vi "4Pi Objective Lock - EMBL_v2.vi"(7 "Calling VI Ref":refnum<vi>) -> ()   [LabVIEW 2021]
uses:
  <vilib>/Utility/miscctls.llb/LVPointTypeDef.ctl
  4Pi Objective Lock Type Defs/4Pi Obj Lock - Notifier Type.ctl
  4Pi Objective Lock Type Defs/4Pi Obj Lock - Actions.ctl
  <vilib>/vision/Image Controls.llb/IMAQ Image.ctl
  4Pi Objective Lock Type Defs/4Pi Obj Lock - Lock Settings.ctl
  Hardware Configuration/Hardware Configuration Controls/Device Type.ctl
  Hardware Configuration/Hardware Configuration Controls/Device Function.ctl
  4Pi Objective Lock Type Defs/4Pi Obj Lock - Camera Settings.ctl
  Device Library/Cameras/Camera Controls/Generic Camera ROI.ctl
  Device Library/Cameras/Camera Controls/Generic Camera Actions.ctl
  Device Library/Stages/Stages Controls/Stage Actions.ctl
  <vilib>/addons/control/pid/pid.llb/PID (DBL Array).vi
  <vilib>/addons/control/pid/pid.llb/PID (DBL).vi
  <vilib>/addons/control/pid/NI_PID_pid.lvlib
  <vilib>/vision/NI_Vision_Development_Module.lvlib
panel:
  out "dz (µm)":dbl format="%.2f"
  out "dxy (px)":dbl[](array[numeric])
  in  "Main Tab":T1(tab)
  out "CC Max Value":dbl=1.0 format="%.3g"
  out "dt z (s)":dbl format="%.3f"
  out "CC Max":cluster{"pixel size (µm)":dbl}(graph)
  out "Z Move":bool
  out "XY Move":bool
  out "Measured X Position (px)":dbl=1.0 format="%.3g"
  out "Measured Y Position (px)":dbl=1.0 format="%.3g"
  out "Measured sx/sy":dbl=1.0 format="%.3g"
  out "Target X Position (px)":dbl=1.0 format="%.3g"
  out "Target Y Position (px)":dbl=1.0 format="%.3g"
  out "Target sx/sy":dbl=1.0 format="%.3g"
  out "Z Axis Position (µm)":dbl=1.0 format="%.4g"
  out "Y Axis Position (µm)":dbl=1.0 format="%.2g"
  out "X Axis Position (µm)":dbl=1.0 format="%.2g"
  out "Z Target and Fit Value (µm)":T2(graph)
  in  "Start Lock":bool
  out "Y Target and Fit Position (µm)":T2(graph)
  out "X Target and Fit Position (µm)":T2(graph)
  in  "Restart Lock":bool
  out "Fit Error":bool
  out "Move Limit Error":bool
  out "Target Z (µm)":dbl=1.0 format="%.3g"
  out "Measured Z (µm)":dbl=1.0 format="%.3g"
  out "Target X Position cc (px)":dbl=1.0 format="%.3g"
  out "Measured X Position cc (px)":dbl=1.0 format="%.3g"
  out "Measured Y Position cc (px)":dbl=1.0 format="%.3g"
  out "Target Y Position cc (px)":dbl=1.0 format="%.3g"
  in  "Metric scale sx/sy":dbl=0.4
  in  "pixel size (µm)":dbl=0.05
  in  "X Update Scale Factor":dbl=0.005
  in  "Y Update Scale Factor":dbl=0.003
  in  "Z Update Scale Factor":dbl=0.4
  in  "Sample Z Step No.":u32=2
  in  "Sample Z Step Size (µm)":dbl=2.0
  in  "Update Delay (ms)":i32=10
  in  "D (Derivative)":dbl
  in  "I (Integral)":dbl
  in  "P (Proportional)":dbl=2.0
  in  "Invert Z Axis":bool
  in  "XY Drift Threshold":dbl=0.05
  in  "Abort If Error":bool
  in  "Flip XY Axis":bool
  in  "Invert X Axis":bool=TRUE
  in  "Invert Y Axis":bool=TRUE
  in  "Z Stage Move Limit (µm)":dbl=5.0
  in  "Z Drift Threshold":dbl=0.05
  in  "XY Stage Move Limit (µm)":dbl=1.0
  in  "Frame Accumulations":u16=10
  in  "XY Correction Active":bool=TRUE
  in  "Z Correction Active":bool=TRUE
  in  "Set Camera ROI":bool
  in  "Save Lock Settings":bool
  in  "Quit":bool
  # "Z Drift Settings"
  # "Camera Setup"
  # "XY Drift Settings"
  # "PID Control Values"
  # "General Settings"
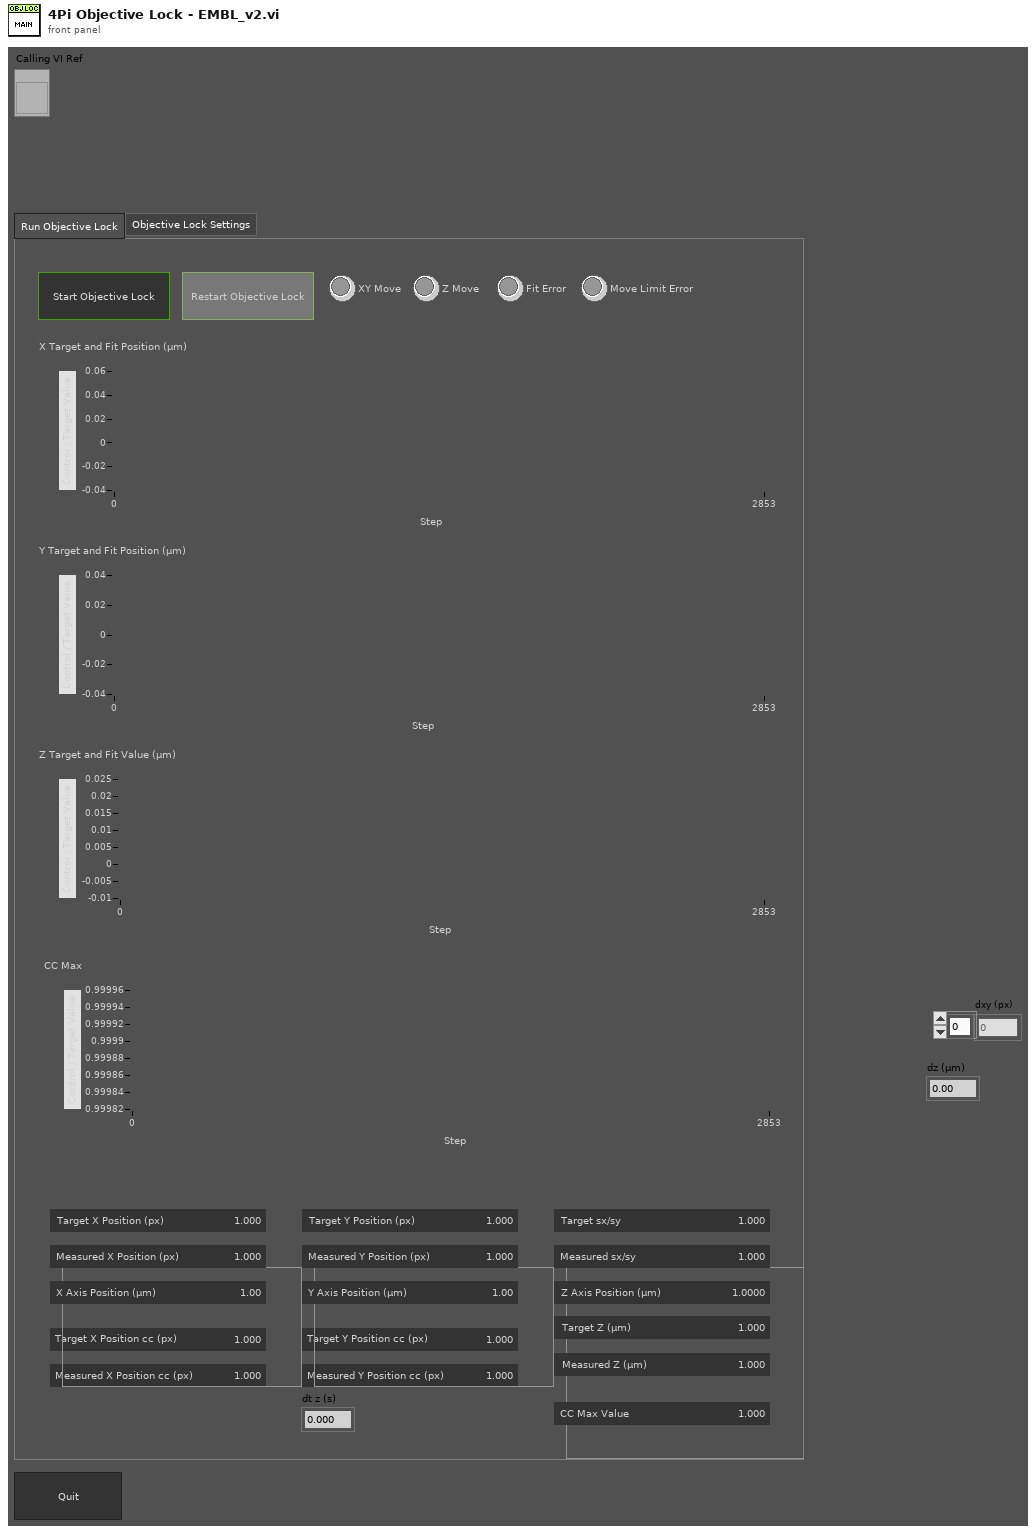
[diagram p1: front panel]
types:
  T1 = enum32{"Run Objective Lock", "Objective Lock Settings"}
  T2 = cluster{"Target 01":dbl, dbl, dbl, "Current 01":dbl, "Stage Pos":dbl, "Current 2":dbl}
  T3 = typedef "4Pi Obj Lock - Camera Settings.ctl" = cluster{"Exposure Time (s)":dbl, "H Offset":u16, "V Offset":u16, "H Width":u16, "V Width":u16}
  T4 = typedef "Device Function.ctl" = enum16{"Primary", "Secondary", "Overview", "Wide Field Drift Correction", "642 nm Excitation", "560 nm Excitation", "940 nm Excitation", "546 nm Excitation", "488 nm Excitation", "405 nm Excitation", "Objective Drift Correction", "4Pi Focus Lock", "4Pi Objective Lock", "Objective XY", "Objective Z", "Sample XY", "Sample Coarse Z", "Sample Z", "4Pi Lower", "4Pi Upper", "Em Small", "Em Large", "Ex Small", "Ex Large", "Mojo", "Adj Cavity", "Line Scanning", "Alert"}
  T5 = typedef "Device Type.ctl" = enum16{"AOTF", "Camera", "Deformable Mirror", "Laser", "Flip Mirror", "Shutter", "Stage", "Waveform", "FPGA", "Email"}
  T6 = typedef "4Pi Obj Lock - Actions.ctl" = enum16{"Idle", "Start Lock", "Restart Lock", "Get Initial Position", "Get Target Z Position", "Get Ref Stack", "Cal Ref FFT", "Move To Init Z", "Get Current Image", "Get Current Z Position", "Get Current XY Position", "Get Current Position", "Check Drift", "Check Drift cc xy", "Check Drift cc z", "Check Drift cc", "Move XYZ", "Move XY", "Move Z", "Update Plots", "Delay", "Abort", "Exit Loop", "Quit"}
  T7 = typedef "4Pi Obj Lock - Lock Settings.ctl" = cluster{"Z Drift Threshold":dbl, "Z Stage Move Limit (µm)":dbl, "XY Drift Threshold":dbl, "XY Stage Move Limit (µm)":dbl, "Frame Accumulations":u16, "Abort If Error":bool, "Flip XY Axis":bool, "Invert X Axis":bool, "Invert Y Axis":bool, "Invert Z Axis":bool, "Z Correction Active":bool, "XY Correction Active":bool, "PID Values":dbl[], "Update Delay (ms)":i32, "Sample Z Step Size (µm)":dbl, "Sample Z Step No.":u32, "Z Update Scale Factor":dbl, "Y Update Scale Factor":dbl, "X Update Scale Factor":dbl}
  T8 = typedef "4Pi Obj Lock - Notifier Type.ctl" = cluster{"Actions":T6, "Z Drift Threshold":dbl, "Z Stage Move Limit (µm)":dbl, "XY Drift Threshold":dbl, "XY Stage Move Limit (µm)":dbl, "Frame Accumulations":u16, "Abort If Error":bool, "Z Correction Active":bool, "XY Correction Active":bool, "PID Values":dbl[], "Running?":bool, "Update Delay (ms)":i32, "Cur Image (SGL)":T9, "Ref Stack (SGL)":T9[], "Sample Z (µm)":dbl[], "Initial Z Position (µm)":dbl, "Z Step Size (µm)":dbl, "Z Step No.":u32, "Ref FFT Stack (CSG)":T9[], "CC Image (SGL) ":T9, "Tmp Image FFT (CSG)":T9[], "CC Image Max (SGL)":T9}
  T9 = typedef "IMAQ Image.ctl" = refnum<image>
  T10 = enum16{"Always On", "Always Off", "Off While Running"}
  T11 = typedef "LVPointTypeDef.ctl" = cluster{"Horizontal":i16, "Vertical":i16}
  T12 = typedef "Image Type" = u32
  T13 = typedef "Generic Camera Actions.ctl" = enum16{"Status", "Live Preview", "Capture", "Abort", "Set Exposure Time (s)", "Get Exposure Time (s)", "Record Settings", "Set ROI", "Get ROI", "Defect Correction On/Off", "Cooler On/Off", "Fan On/Off", "Quit"}
  T14 = typedef "Generic Camera ROI.ctl" = cluster{"H_Offset":u16, "V_Offset":u16, "H_Width":u16, "V_Width":u16}
  T15 = typedef "Stage Actions.ctl" = enum16{"Get Position", "SERVO OFF", "SERVO ON", "SERVO ON/OFF", "MVR", "MOVE", "HALT", "ONTARGET", "ERROR", "REFERENCE", "INIT", "VELOCITY", "STATUS", "EXIT", "HOME", "ZEROPOS", "NANOPOS", "ANALOG", "QUIT"}
  T16 = enum32{"Invalid", "Standard", "Closed", "Hidden", "Minimized", "Maximized"}
  T17 = cluster{"Target 01":dbl, dbl, dbl, "Current 01":dbl, "Stage Pos":dbl, "Current 2":dbl}[]
  T18 = typedef "Stage Status.ctl" = enum16{"Error", "Abort", "Busy", "On Target"}
  T19 = typedef "2D Gaussian - Best Fit Parameters.ctl" = cluster{"Amplitude":dbl, "X Position":dbl, "Y Position":dbl, "X Width":dbl, "Y Width":dbl, "Offset":dbl}
  T20 = cluster{"PID Values[0]":dbl, "PID Values[1]":dbl, "PID Values[2]":dbl}
  T21 = cluster{"PID Values[0]":dbl, "PID Values[1]":dbl, "PID Values[2]":dbl}[]
  T22 = typedef "LVRectTypeDef.ctl" = cluster{"Left":i16, "Top":i16, "Right":i16, "Bottom":i16}
  T23 = typedef "LVBoundsTypeDef.ctl" = cluster{"Width":u32, "Height":u32}
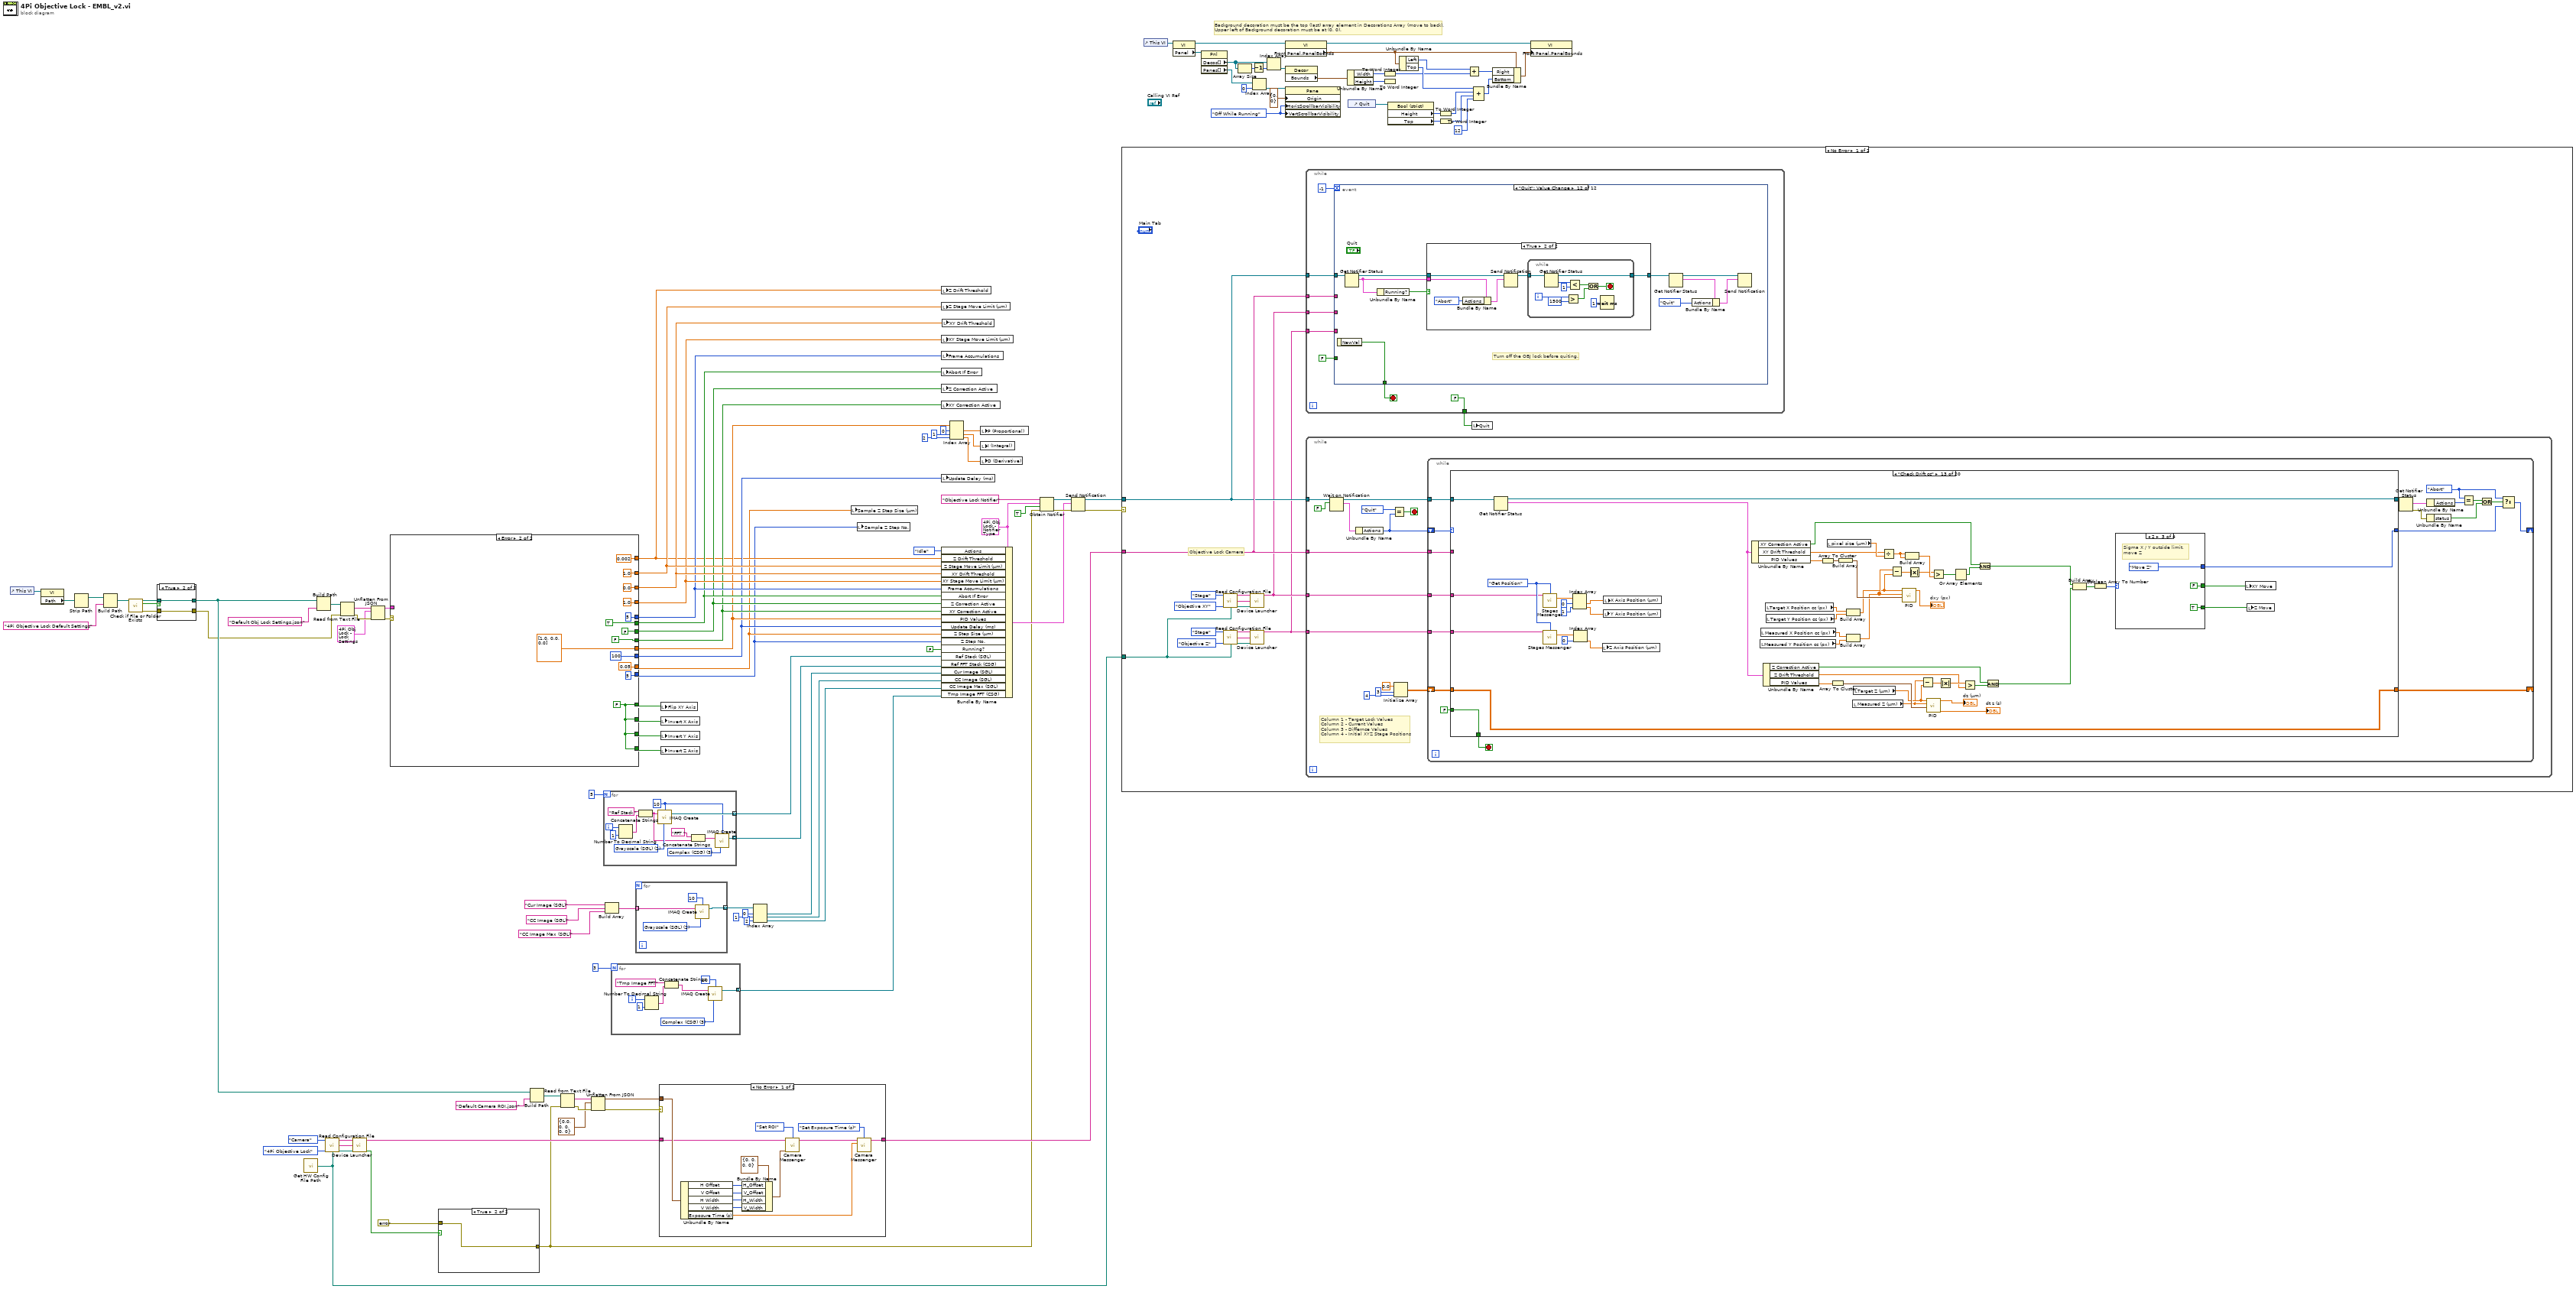
[diagram p0: block diagram]
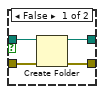
[diagram p2: hidden frame]
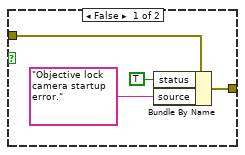
[diagram p3: hidden frame]
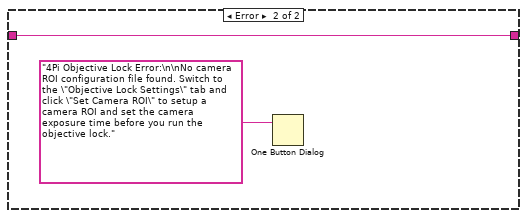
[diagram p4: hidden frame]
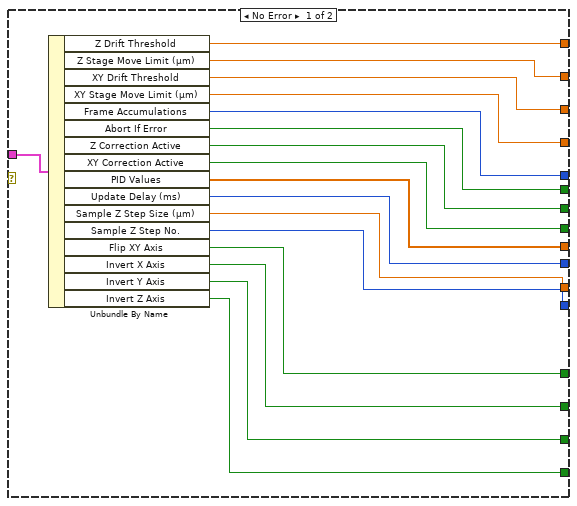
[diagram p5: hidden frame]
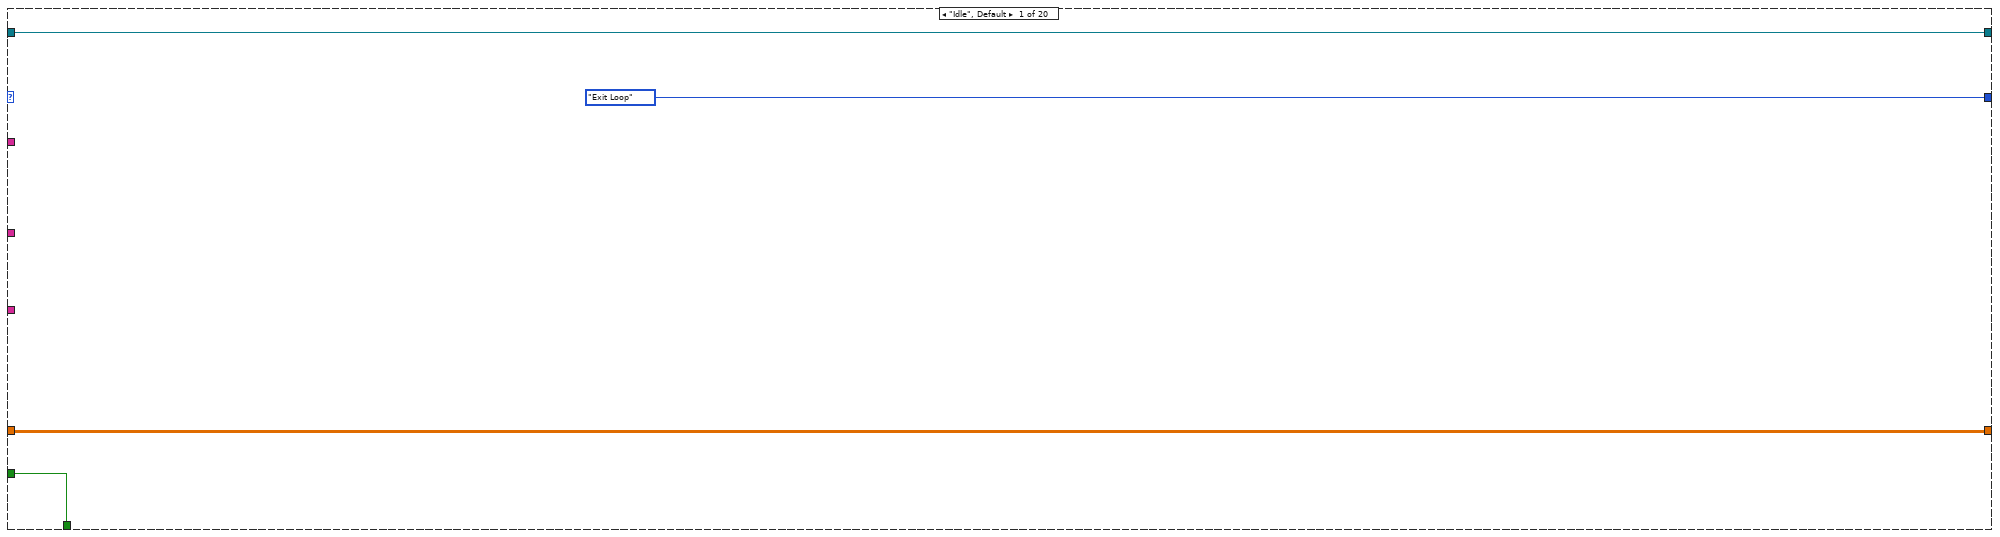
[diagram p6: hidden frame]
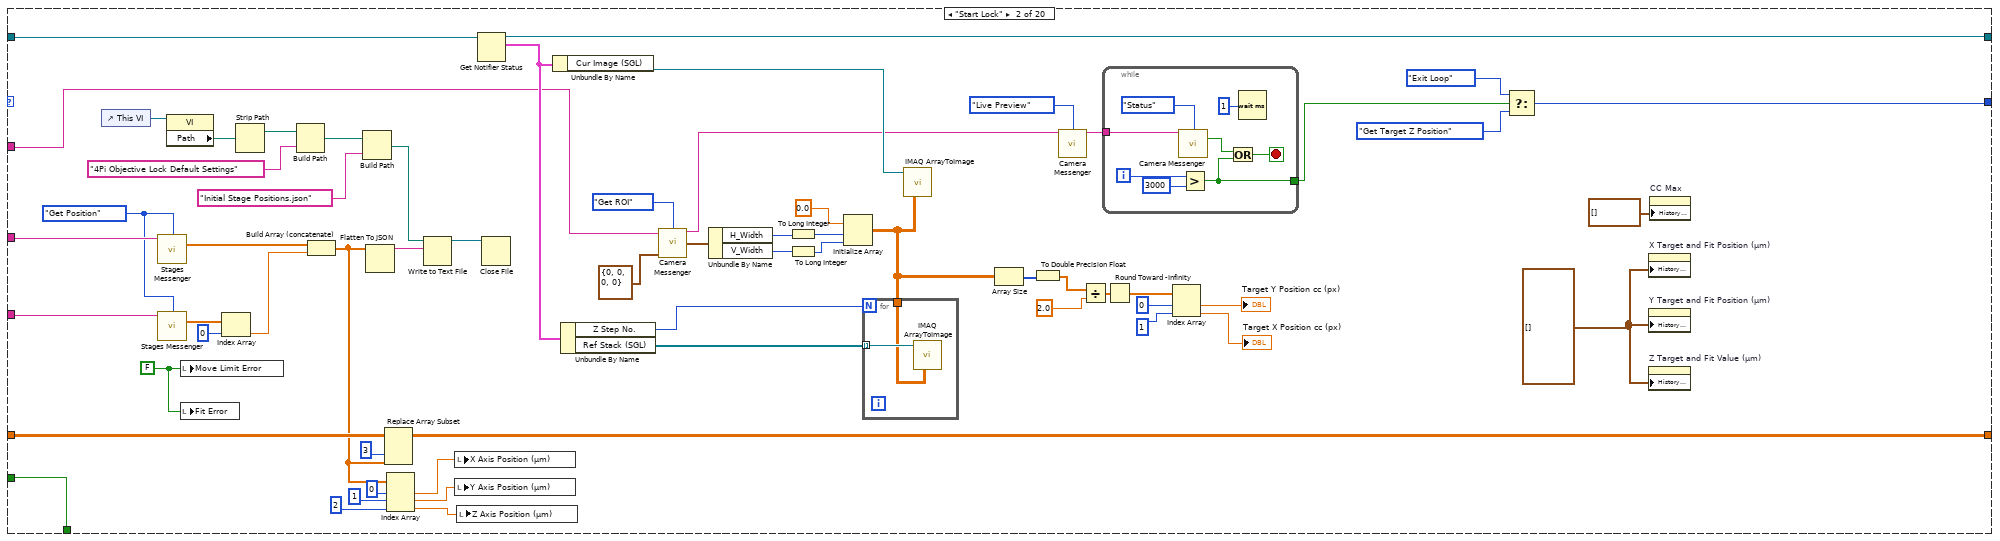
[diagram p7: hidden frame]
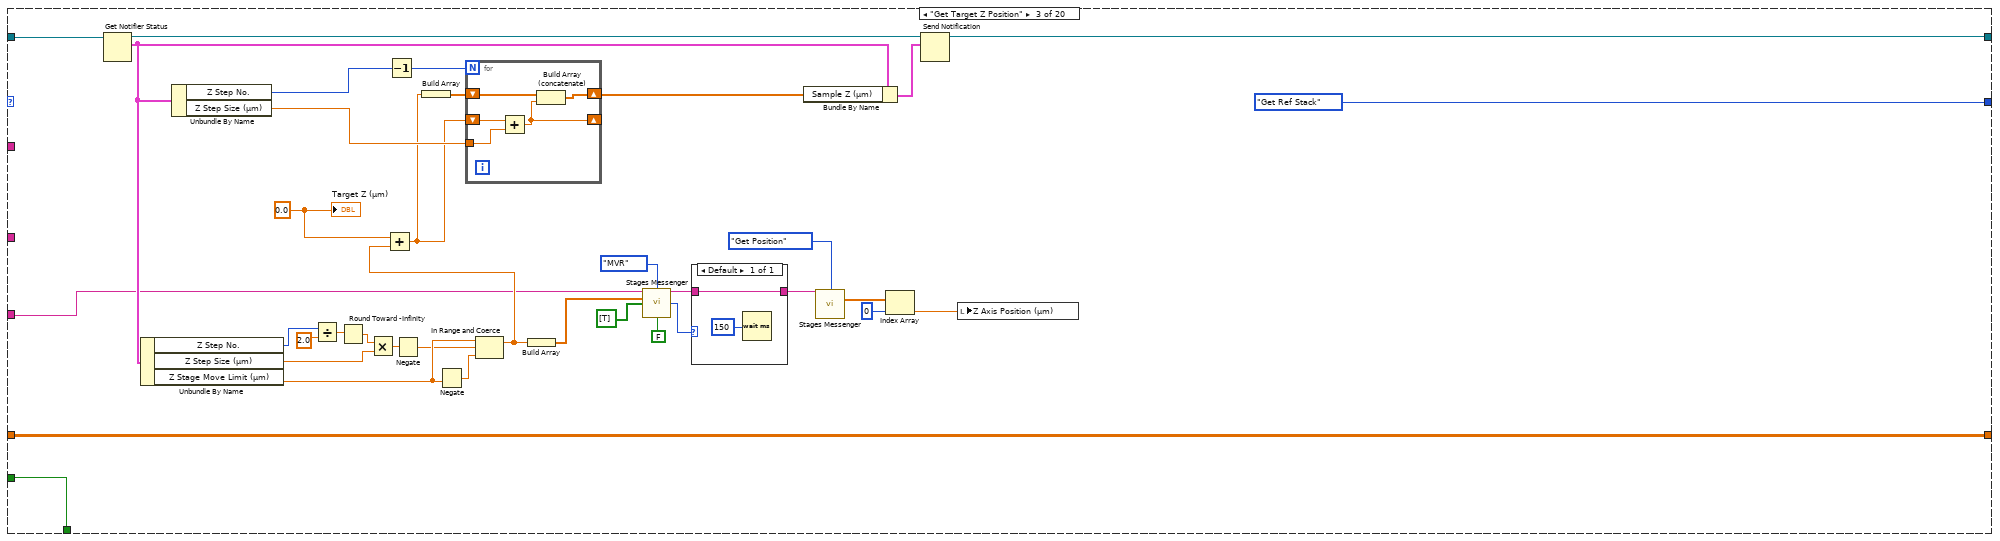
[diagram p8: hidden frame]
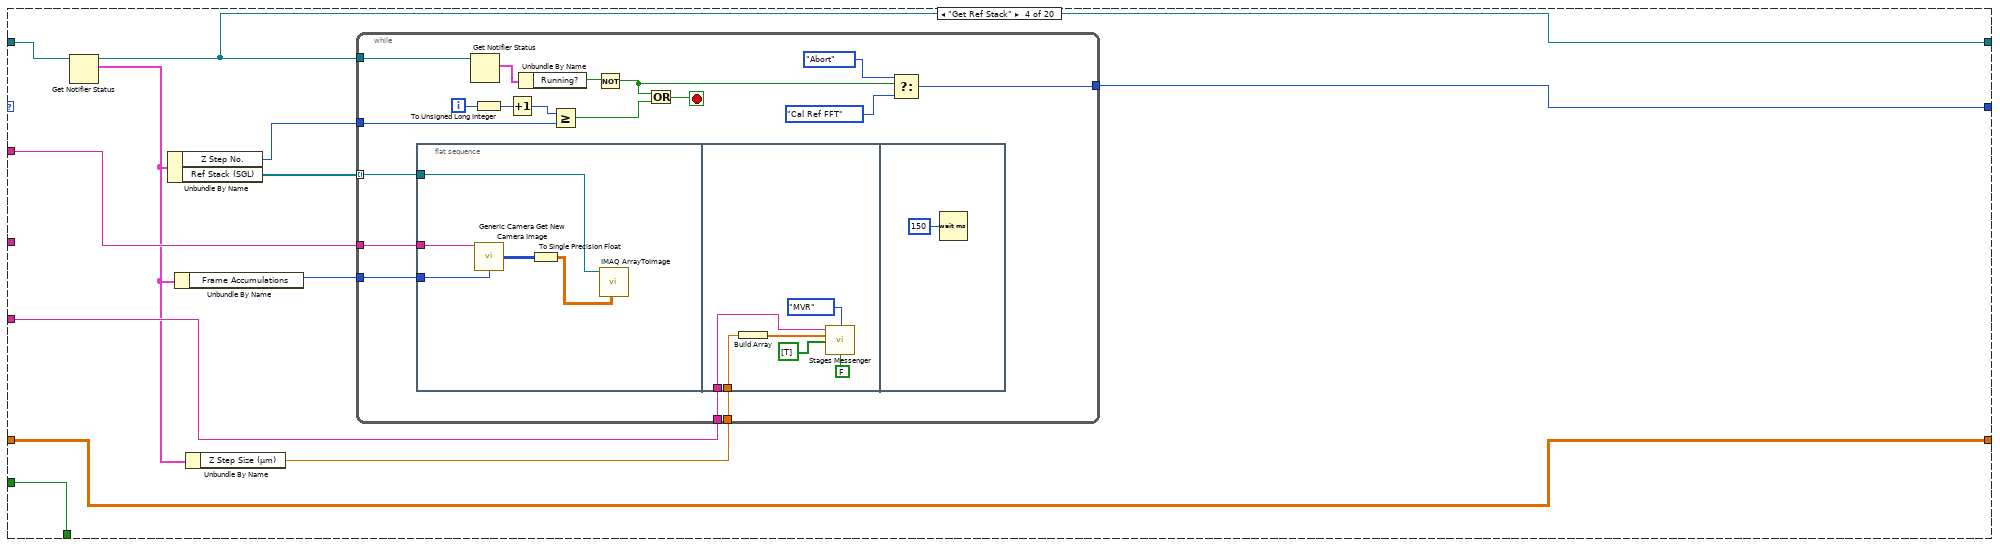
[diagram p9: hidden frame]
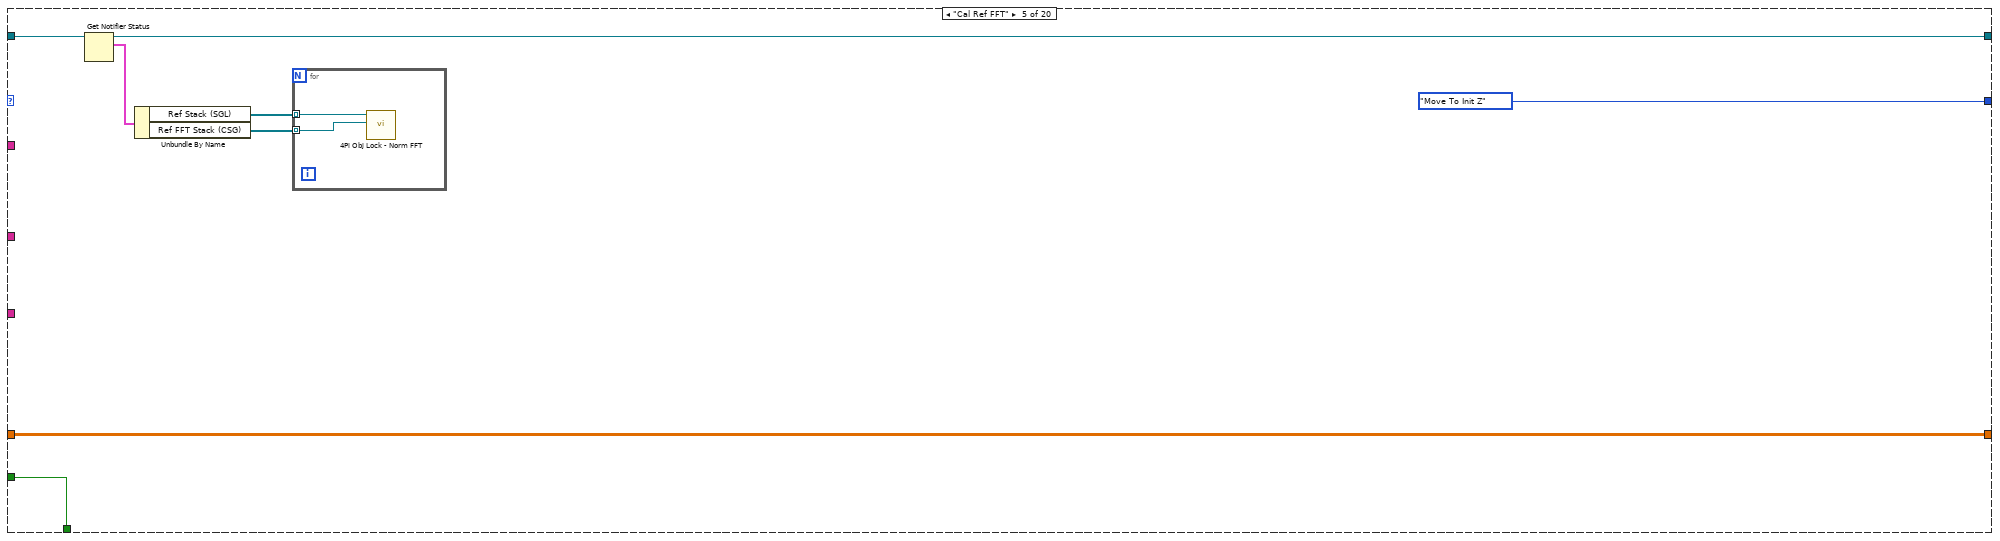
[diagram p10: hidden frame]
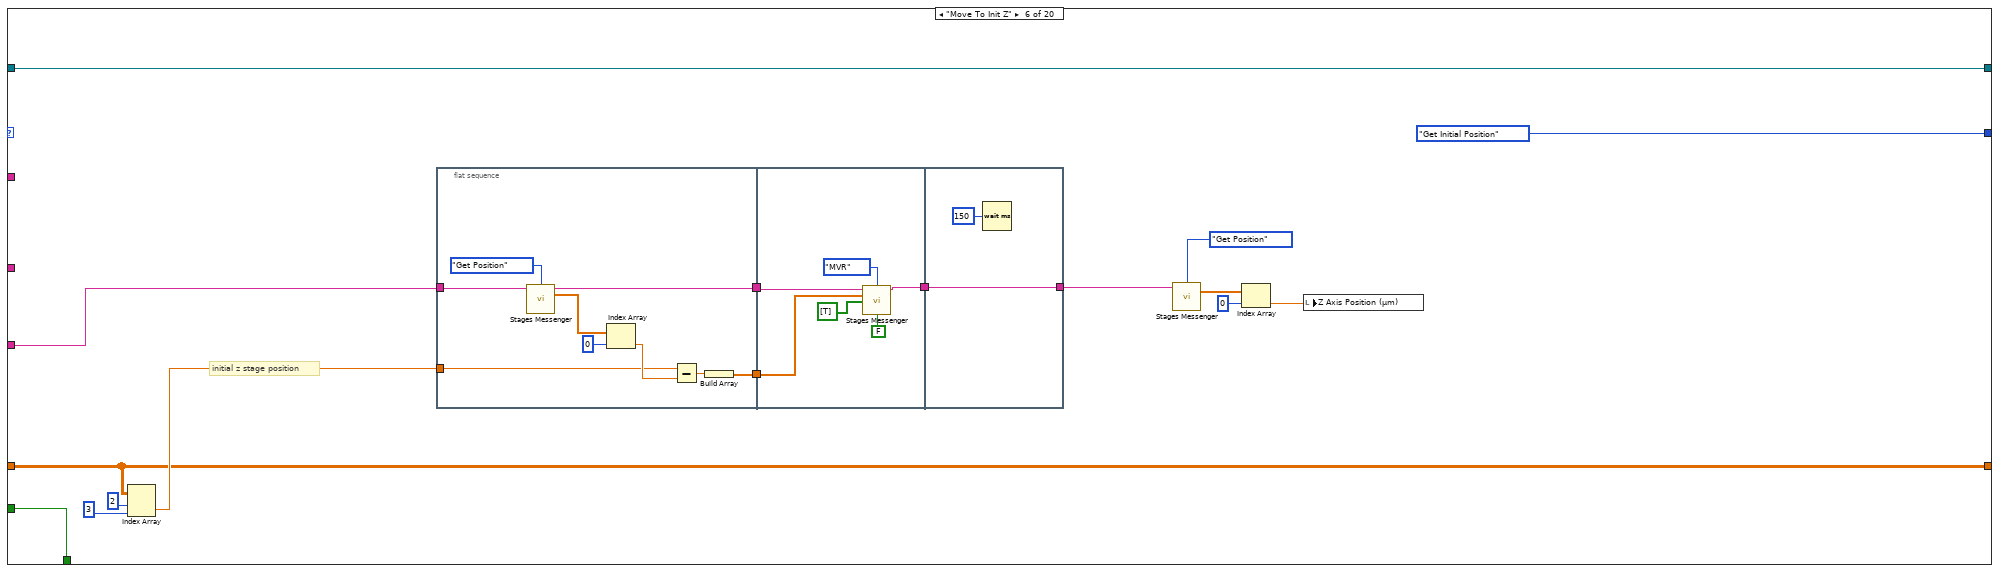
[diagram p11: hidden frame]
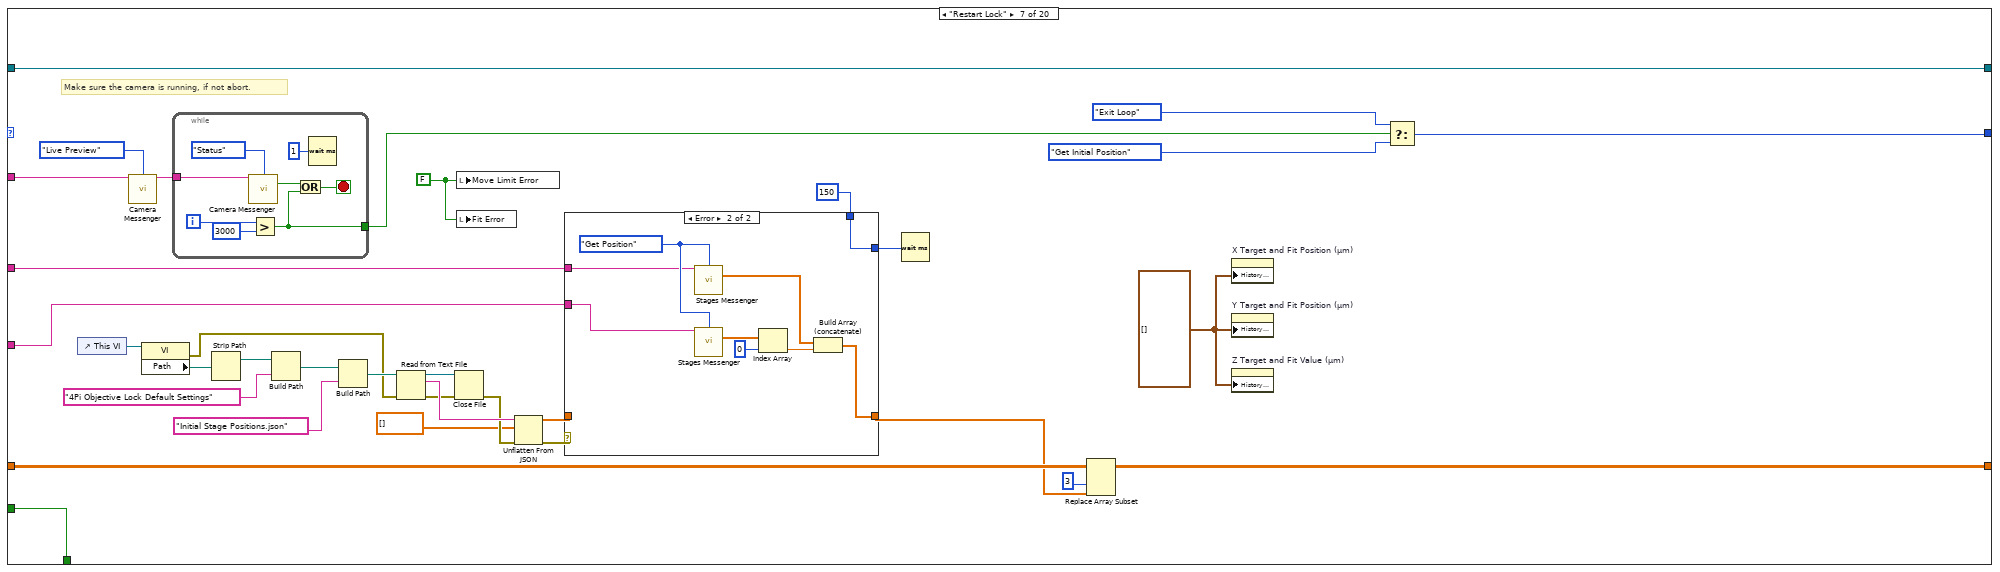
[diagram p12: hidden frame]
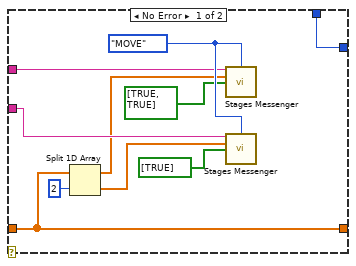
[diagram p13: hidden frame]
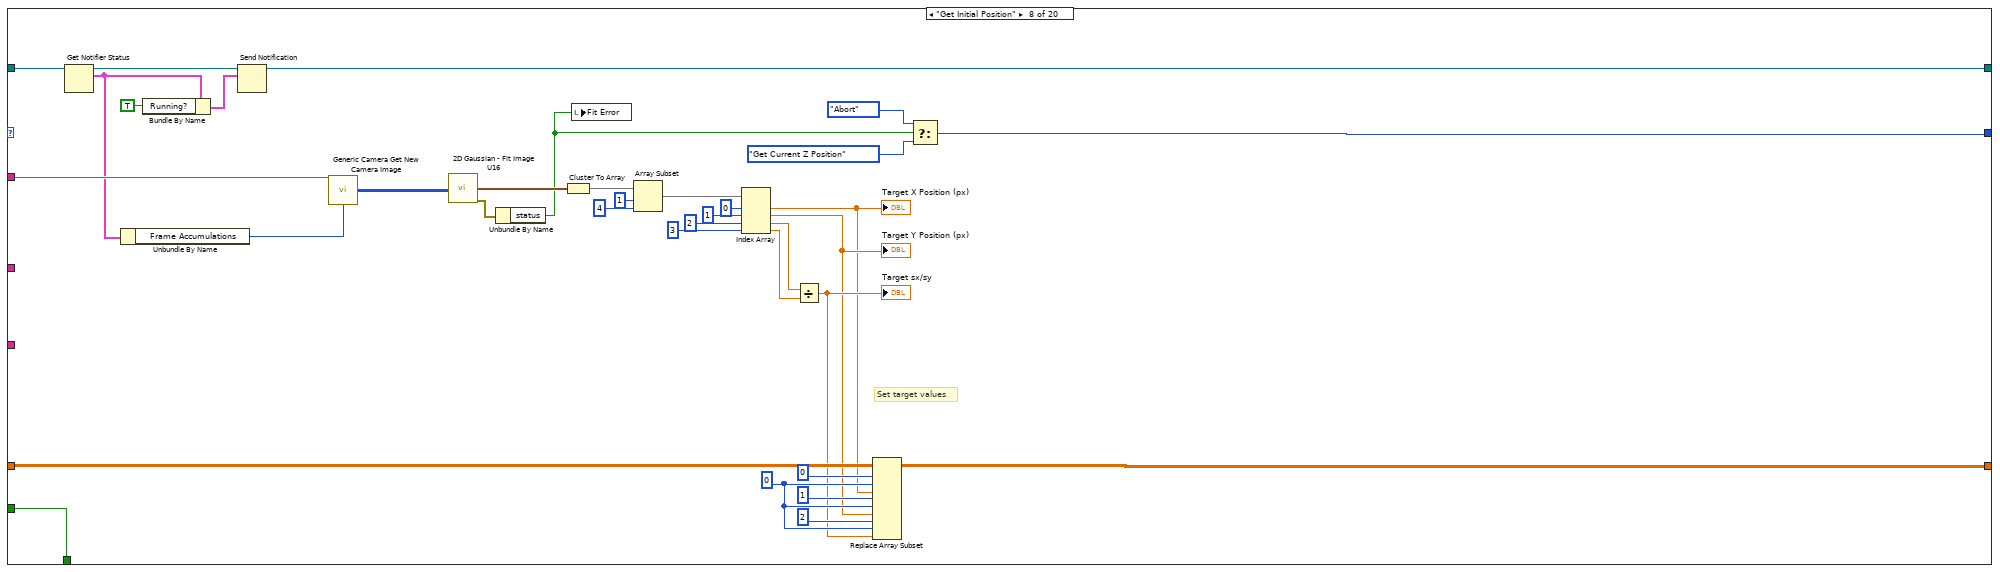
[diagram p14: hidden frame]
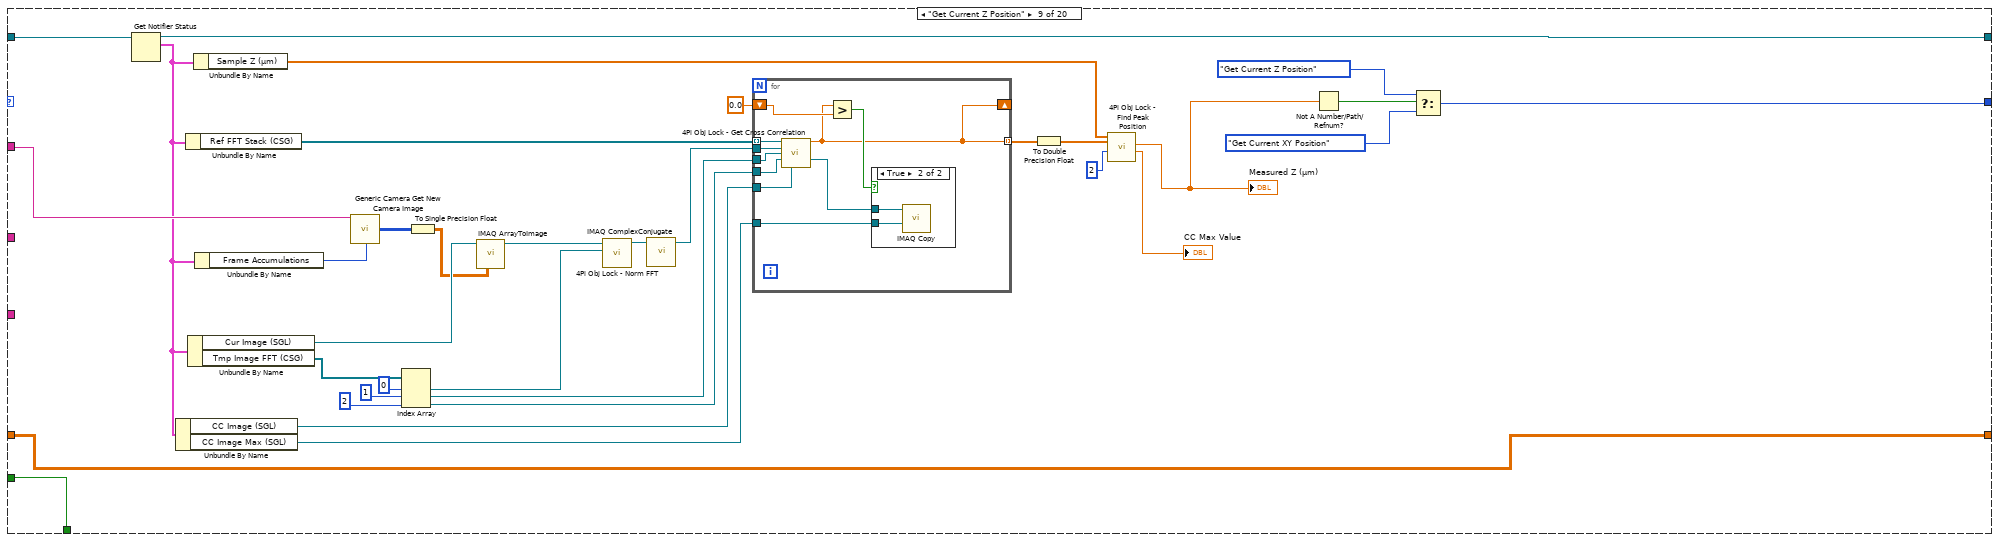
[diagram p15: hidden frame]
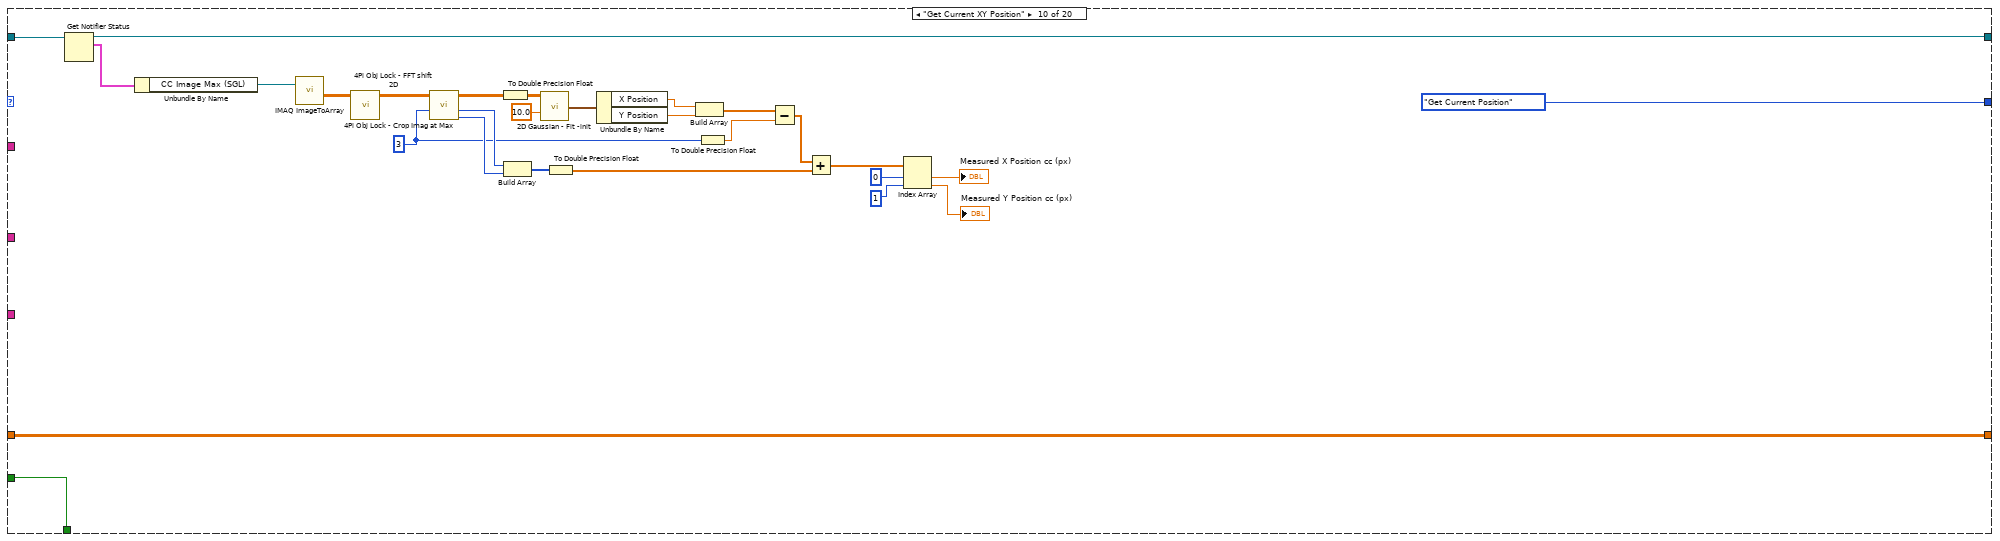
[diagram p17: hidden frame]
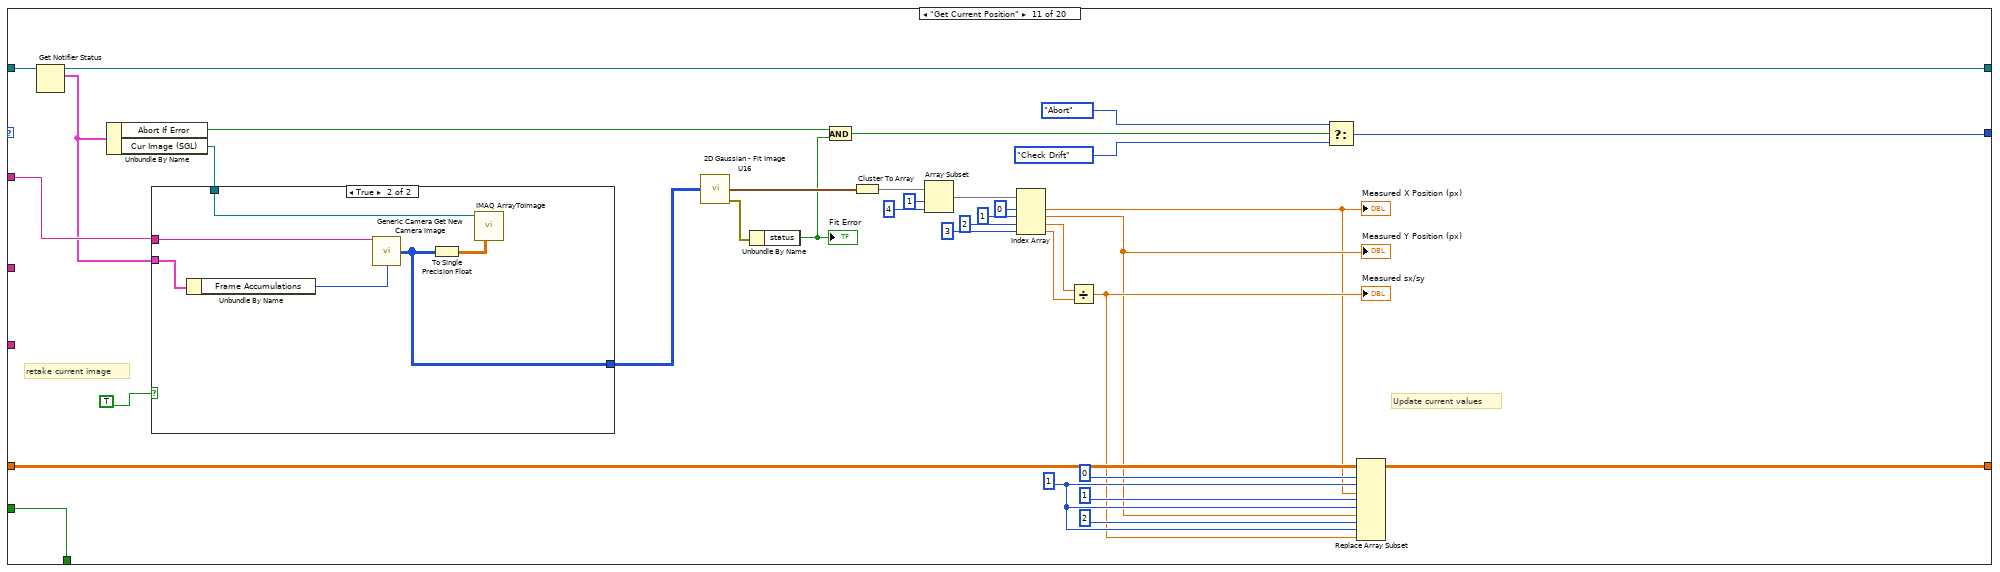
[diagram p18: hidden frame]
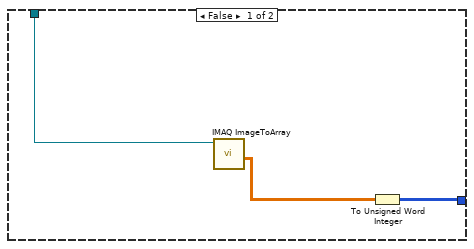
[diagram p19: hidden frame]
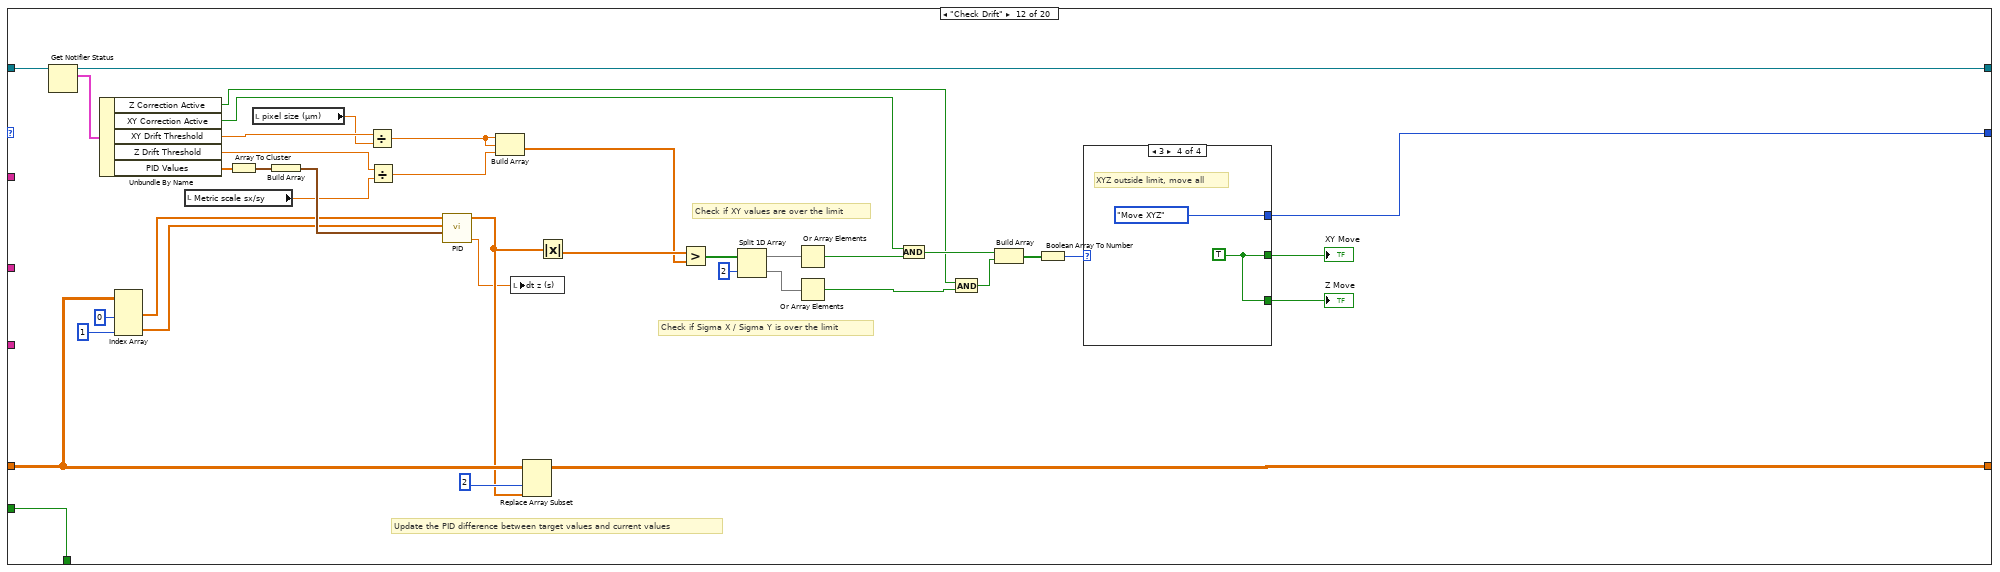
[diagram p20: hidden frame]
diagram:
  w78 = T8 {"Actions"=enum."Idle", "Z Drift Threshold"=0.05, "Z Stage Move Limit (µm)"=1.0, "XY Drift Threshold"=0.05, "XY Stage Move Limit (µm)"=1.0, "Frame Accumulations"=10, "Abort If Error"=FALSE, "Z Correction Active"=FALSE, "XY Correction Active"=FALSE, "PID Values"=[], "Running?"=FALSE, "Update Delay (ms)"=0, "Cur Image (SGL)"=refnum, "Ref Stack (SGL)"=[], "Sample Z (µm)"=[], "Initial Z Position (µm)"=0.0, "Z Step Size (µm)"=2.0, "Z Step No."=2, "Ref FFT Stack (CSG)"=[], "CC Image (SGL) "=refnum, "Tmp Image FFT (CSG)"=[], "CC Image Max (SGL)"=refnum} ("4Pi Obj Lock")
  w95 = T10."Off While Running" ("Vertical Scrollbar Visibility")
  # "Background decoration must be the top (last) array element in Decorations Array (move to back).\nUpper left of Background decoration must be at (0, 0)."
  n1 = control-ref of="This VI"() -> (w66:refnum<vi>)
  n2 = property class="VI"(reference=w66) -> ("Path"=w48:path)  [unwired: 1 in, 2 out]
  n3 = Strip Path(path=w48) -> (stripped path=w47:path)  [unwired: 1 out]
  n4 = Build Path(base path=w47, name or relative path="4Pi Objective Lock Default Settings") -> (appended path=w24:path)
  n5 = call <vilib>:"Check if File or Folder Exists.vi"("path"=w24) -> ("error out"=w20:errorcluster, "file or folder exists?"=w23:bool, "dup path"=w22:path)  [unwired: 8 in]
  n6 = case shown="True" w23 {
    tunnel: w22 -> [w116 w118]
    tunnel: [w115 w118] -> w21
    tunnel: w20 -> [w114 w117]
    tunnel: [w113 w117] -> w19
    frame False {
      n7 = Create Folder(path (use dialog)=w116, error in=w114) -> (created path=w115:path, error out=w113:errorcluster)  [unwired: 1 in, 1 out]
    }
    frame True {
    }
  }
  n8 = call "Get HW Config File Path.vi"() -> ("File Path"=w56:path)  [unwired: 14 in, 1 out]
  n9 = Build Path(base path=w21, name or relative path="Default Obj Lock Settings.json") -> (appended path=w75:path)
  n10 = call "Read Configuration File.vi"("Device Type"=Device_Type."Camera", "Device Function"=Device_Function."4Pi Objective Lock", "Config File Path"=w56) -> ("Unique Notifier Name"=w63:string, "Device Ports/IDs/Channels"=w65:string[], "Device Engine Path"=w64:path)  [unwired: 9 in, 1 out]
  n11 = Read from Text File(file (use dialog)=w75, error in=w19) -> (text=w74:string, error out=w73:errorcluster)  [unwired: 2 in, 2 out]
  n12 = call "Device Launcher.vi"("Notifier Name"=w63, "Device Ports/IDs/Channels"=w65, "Device Engine Path"=w64) -> ("Notifier Name"=w54:string, "Running?"=w60:bool)  [unwired: 11 in]
  n13 = Unflatten From JSON(JSON string=w74, type and defaults=T7 {"Z Drift Threshold"=0.05, "Z Stage Move Limit (µm)"=1.0, "XY Drift Threshold"=0.05, "XY Stage Move Limit (µm)"=1.0, "Frame Accumulations"=10, "Abort If Error"=FALSE, "Flip XY Axis"=FALSE, "Invert X Axis"=FALSE, "Invert Y Axis"=FALSE, "Invert Z Axis"=FALSE, "Z Correction Active"=TRUE, "XY Correction Active"=TRUE, "PID Values"=[], "Update Delay (ms)"=0, "Sample Z Step Size (µm)"=2.0, "Sample Z Step No."=2, "Z Update Scale Factor"=2.0, "Y Update Scale Factor"=2.0, "X Update Scale Factor"=2.0} ("Lock Settings"), error in (no error)=w73) -> (value=w70:T7, error out=w71:errorcluster)  [unwired: 4 in]
  n14 = case shown="Error" w71 {
    tunnel: [w134 0.002 ("Z Drift Threshold")] -> w25
    tunnel: [w133 1.0 ("Z Stage Move Limit (µm)")] -> w40
    tunnel: [w131 0.0 ("XY Drift Threshold")] -> w39
    tunnel: [w132 1.0 ("XY Stage Move Limit (µm)")] -> w38
    tunnel: [w130 u16 5 ("Frame Accumulations")] -> w37
    tunnel: [w129 TRUE ("Abort If Error")] -> w36
    tunnel: w70 -> [w135 _]
    tunnel: [w128 FALSE ("Z Correction Active")] -> w35
    tunnel: [w127 FALSE ("XY Correction Active")] -> w34
    tunnel: [w126 dbl[] [1.0, 0.0, 0.0] ("PID Values")] -> w33
    tunnel: [w125 u16 100 ("Update Delay (ms)")] -> w26
    tunnel: [w124 w138] -> w42
    tunnel: [w123 w138] -> w43
    tunnel: [w122 w138] -> w44
    tunnel: [w121 w138] -> w45
    tunnel: [w120 0.05 ("Sample Z Step Size (µm)")] -> w5
    tunnel: [w119 u32 5 ("Sample Z Step No.")] -> w4
    frame No Error {
      n15 = Unbundle By Name(w135) -> ("Z Drift Threshold"=w134:dbl, "Z Stage Move Limit (µm)"=w133:dbl, "XY Drift Threshold"=w131:dbl, "XY Stage Move Limit (µm)"=w132:dbl, "Frame Accumulations"=w130:u16, "Abort If Error"=w129:bool, "Z Correction Active"=w128:bool, "XY Correction Active"=w127:bool, "PID Values"=w126:dbl[], "Update Delay (ms)"=w125:i32, "Sample Z Step Size (µm)"=w120:dbl, "Sample Z Step No."=w119:u32, "Flip XY Axis"=w121:bool, "Invert X Axis"=w122:bool, "Invert Y Axis"=w123:bool, "Invert Z Axis"=w124:bool)
    }
    frame Error {
      w138 = FALSE ("Flip XY Axis")
    }
  }
  n16 = case shown="True" w60 {
    tunnel: errorcluster {"status"=FALSE, "code"=0, "source"=""} ("Error") -> [w152 w153]
    tunnel: [w149 w153] -> w46
    frame False {
      n17 = Bundle By Name(cluster=w152, "status"=TRUE, "source"="Objective lock camera startup error." ("name or relative path")) -> (w149:errorcluster)
    }
    frame True {
    }
  }
  n18 = Build Path(base path=w21, name or relative path="Default Camera ROI.json") -> (appended path=w50:path)
  n19 = Read from Text File(file (use dialog)=w50, error in=w46) -> (text=w68:string, error out=w67:errorcluster)  [unwired: 2 in, 2 out]
  n20 = Unflatten From JSON(JSON string=w68, type and defaults=T3 {"Exposure Time (s)"=0.0, "H Offset"=0, "V Offset"=0, "H Width"=0, "V Width"=0} ("Camera Settings"), error in (no error)=w67) -> (value=w53:T3, error out=w58:errorcluster)  [unwired: 4 in]
  n21 = for {
    N: 5 -> [_]
    tunnel: [w165] -> w17 mode=indexing
    tunnel: [w154] -> w16 mode=indexing
    i -> [w164]
    w159 = T12 3 items=["Grayscale (U8)", "Grayscale (I16)", "Grayscale (SGL)", "Complex (CSG)", "RGB (U32)", "HSL (U32)", "RGB (U64)", "Grayscale (U16)"] ("Image Type")
    w160 = T12 2 items=["Grayscale (U8)", "Grayscale (I16)", "Grayscale (SGL)", "Complex (CSG)", "RGB (U32)", "HSL (U32)", "RGB (U64)", "Grayscale (U16)"] ("Image Type")
    w156 = 10 ("Border Size")
    n22 = Number To Decimal String(number=w164, width (-)=i16 1) -> (decimal integer string=w162:string)
    n23 = Concatenate Strings("Ref Stack " ("string"), w162) -> (w155:string)
    n24 = call "IMAQ Create"("Border Size"=w156, "Image Name"=w155, "Image Type"=w160) -> ("New Image"=w165:T9)  [unwired: 2 in, 1 out]
    n25 = Concatenate Strings("FFT " ("string"), w155) -> (w158:string)
    n26 = call "IMAQ Create"("Border Size"=w156, "Image Name"=w158, "Image Type"=w159) -> ("New Image"=w154:T9)  [unwired: 2 in, 1 out]
  }
  n27 = Build Array("Cur Image (SGL)" ("Image Name"), "CC Image (SGL)" ("Image Name"), "CC Image Max (SGL)" ("Image Name")) -> (w11:string[])
  n28 = for {
    N: 3 -> [_]
    tunnel: [w171] -> w6 mode=indexing
    i -> [w167]
    w172 = T12 3 items=["Grayscale (U8)", "Grayscale (I16)", "Grayscale (SGL)", "Complex (CSG)", "RGB (U32)", "HSL (U32)", "RGB (U64)", "Grayscale (U16)"] ("Image Type")
    n29 = Number To Decimal String(number=w167, width (-)=i16 1) -> (decimal integer string=w170:string)
    n30 = Concatenate Strings("Tmp Image FFT" ("Image Name"), w170) -> (w166:string)
    n31 = call "IMAQ Create"("Border Size"=10, "Image Name"=w166, "Image Type"=w172) -> ("New Image"=w171:T9)  [unwired: 2 in, 1 out]
  }
  n32 = for {
    tunnel: w11 -> [w175] mode=indexing
    tunnel: [w174] -> w10 mode=indexing
    w176 = T12 2 items=["Grayscale (U8)", "Grayscale (I16)", "Grayscale (SGL)", "Complex (CSG)", "RGB (U32)", "HSL (U32)", "RGB (U64)", "Grayscale (U16)"] ("Image Type")
    n33 = call "IMAQ Create"("Border Size"=10, "Image Name"=w175, "Image Type"=w176) -> ("New Image"=w174:T9)  [unwired: 2 in, 1 out]
  }
  n34 = case shown="No Error" w58 {
    tunnel: w54 -> [w181 w192]
    tunnel: w53 -> [w190 _]
    tunnel: [w178 w192] -> w52
    frame No Error {
      n35 = Unbundle By Name(w190) -> ("H Offset"=w185:u16, "V Offset"=w186:u16, "H Width"=w187:u16, "V Width"=w188:u16, "Exposure Time (s)"=w180:dbl)
      n36 = Bundle By Name(cluster=T14 {"H_Offset"=0, "V_Offset"=0, "H_Width"=0, "V_Width"=0} ("General Camera ROI"), "H_Offset"=w185, "V_Offset"=w186, "H_Width"=w187, "V_Width"=w188) -> (w184:T14)
      n37 = call "Camera Messenger.vi"("Notifier Name"=w181, "General Camera Actions"=Generic_Camera_Actions."Set ROI", "Camera ROI"=w184) -> ("Notifier Name Dup"=w179:string)  [unwired: 7 in, 5 out]
      n38 = call "Camera Messenger.vi"("Notifier Name"=w179, "General Camera Actions"=Generic_Camera_Actions."Set Exposure Time (s)", "Exposure Time (s)"=w180) -> ("Notifier Name Dup"=w178:string)  [unwired: 7 in, 5 out]
    }
    frame Error {
      n39 = One Button Dialog(message="4Pi Objective Lock Error:\n\nNo camera ROI configuration file found. Switch to the \"Objective Lock Settings\" tab and click \"Set Camera ROI\" to setup a camera ROI and set the camera exposure time before you run the objective lock.") -> ()  [unwired: 1 in, 1 out]
    }
  }
  n40 = local write "Flip XY Axis"(w45) -> ()
  n41 = local write "Invert X Axis"(w44) -> ()
  n42 = local write "Invert Y Axis"(w43) -> ()
  n43 = local write "Invert Z Axis"(w42) -> ()
  n44 = Index Array(array=w10, index #1=0 ("index"), index #2=1 ("index"), index #3=2 ("index")) -> (element #1=w9:T9, element #2=w8:T9, element #3=w1:T9)
  n45 = local write "Sample Z Step Size (µm)"(w5) -> ()
  n46 = local write "Sample Z Step No."(w4) -> ()
  n47 = Bundle By Name(cluster=w78, "Actions"=4Pi_Obj_Lock_-_Actions."Idle", "Z Drift Threshold"=w25, "Z Stage Move Limit (µm)"=w40, "XY Drift Threshold"=w39, "XY Stage Move Limit (µm)"=w38, "Frame Accumulations"=w37, "Abort If Error"=w36, "Z Correction Active"=w35, "XY Correction Active"=w34, "PID Values"=w33, "Update Delay (ms)"=w26, "Z Step Size (µm)"=w5, "Z Step No."=w4, "Running?"=FALSE ("Obj Lock Active?"), "Ref Stack (SGL)"=w17, "Ref FFT Stack (CSG)"=w16, "Cur Image (SGL)"=w9, "CC Image (SGL)"=w8, "CC Image Max (SGL)"=w1, "Tmp Image FFT (CSG)"=w6) -> (w77:T8)
  n48 = local write "Z Drift Threshold"(w25) -> ()
  n49 = local write "Z Stage Move Limit (µm)"(w40) -> ()
  n50 = local write "XY Stage Move Limit (µm)"(w38) -> ()
  n51 = local write "Frame Accumulations"(w37) -> ()
  n52 = local write "Abort If Error"(w36) -> ()
  n53 = local write "Z Correction Active"(w35) -> ()
  n54 = local write "XY Correction Active"(w34) -> ()
  n55 = local write "Update Delay (ms)"(w26) -> ()
  n56 = local write "XY Drift Threshold"(w39) -> ()
  n57 = Index Array(array=w33, index #1=0 ("index"), index #2=1 ("index"), index #3=2 ("index")) -> (element #1=w29:dbl, element #2=w27:dbl, element #3=w28:dbl)
  n58 = local write "P (Proportional)"(w29) -> ()
  n59 = local write "I (Integral)"(w27) -> ()
  n60 = local write "D (Derivative)"(w28) -> ()
  n61 = Obtain Notifier(name (unnamed)="Objective Lock Notifier", notification data type=w78, create if not found? (T)=TRUE, error in (no error)=w46) -> (notifier out=w80:refnum<notifier>, error out=w81:errorcluster)  [unwired: 1 out]
  n62 = Send Notification(notification=w77, notifier=w80, error in (no error)=w81) -> (notifier out=w79:refnum<notifier>, error out=w57:errorcluster)
  n63 = case shown="No Error" w57 {
    tunnel: w56 -> [w197 _]
    tunnel: w79 -> [w195 _]
    tunnel: w52 -> [w196 _]
    frame No Error {
      # "Objective Lock Camera"
      n64 = call "Read Configuration File.vi"("Device Type"=Device_Type."Stage", "Device Function"=Device_Function."Objective XY", "Config File Path"=w197) -> ("Unique Notifier Name"=w205:string, "Device Ports/IDs/Channels"=w203:string[], "Device Engine Path"=w204:path)  [unwired: 9 in, 1 out]
      n65 = call "Read Configuration File.vi"("Device Type"=Device_Type."Stage", "Device Function"=Device_Function."Objective Z", "Config File Path"=w197) -> ("Unique Notifier Name"=w200:string, "Device Ports/IDs/Channels"=w202:string[], "Device Engine Path"=w201:path)  [unwired: 9 in, 1 out]
      n66 = call "Device Launcher.vi"("Notifier Name"=w205, "Device Ports/IDs/Channels"=w203, "Device Engine Path"=w204) -> ("Notifier Name"=w194:string)  [unwired: 11 in, 1 out]
      n67 = call "Device Launcher.vi"("Notifier Name"=w200, "Device Ports/IDs/Channels"=w202, "Device Engine Path"=w201) -> ("Notifier Name"=w193:string)  [unwired: 11 in, 1 out]
      n68 = while {
        tunnel: [FALSE] -> w208
        tunnel: w196 -> [w1066]
        tunnel: w195 -> [w1065]
        tunnel: w194 -> [w1064]
        tunnel: w193 -> [w1063]
        stop <- w1068 stop-if-true
        n69 = event shown="[11] \"Quit\": Value Change" {
          selector: _ -> [_ _ _ _ _ _ _ _ _ _ _ _]
          dyn-events: _ -> [_ _ _ _ _ _ _ _ _ _ _ _]
          timeout: -1 -> [_ _ _ _ _ _ _ _ _ _ _ _]
          tunnel: FALSE -> [w1071 w1075 w1078 w1088 w1108 w1143 w1170 w1177 w1206 w1216 w1223 _]
          tunnel: [w1071 w1075 w1078 w1088 w1108 w1143 w1170 w1177 w1206 w1216 w1223 w1233] -> w1068
          tunnel: w1066 -> [_ _ w1077 _ _ _ _ _ _ _ _ _]
          tunnel: w1065 -> [_ _ _ w1087 w1105 w1146 w1169 w1176 w1205 w1215 w1222 w1228]
          tunnel: w1064 -> [_ _ _ _ _ _ _ _ _ _ _ _]
          tunnel: w1063 -> [_ _ _ _ _ _ _ _ _ _ _ _]
          event Timeout {
            n70 = event-data() -> ()  [unwired: 1 in, 1 out]
          }
          event Application Instance Close? {
            n71 = event-data() -> ()  [unwired: 1 in, 1 out]
            n72 = control-ref of="This VI"() -> (w1072:refnum<vi>)
            n73 = invoke class="VI" method="FP.Open"(reference=w1072, "Activate"=TRUE ("Activate?"), "State"=T16."Standard") -> ()  [unwired: 2 in, 5 out]
            n74 = event-data("Discard?"=TRUE) -> ()  [unwired: 1 in, 1 out]
          }
          event "Set Camera ROI": Value Change {
            n75 = event-data() -> ()  [unwired: 1 in, 2 out]
            n76 = call "4Pi Obj Lock - Setup Camera.vi"("Camera Notifier Name"=w1077) -> ()  [unwired: 14 in, 1 out]
          }
          event "XY Correction Active", "Z Correction Active", "Abort If Error": Value Change {
            n77 = event-data() -> ("NewVal"=w1083:bool, "CtlRef"=w1086:refnum<vi>)  [unwired: 1 in]
            n78 = Get Notifier Status(notifier=w1087) -> (notifier out=w1085:refnum<notifier>, current notification=w1082:T8)  [unwired: 1 in, 3 out]
            n79 = property class="Bool (strict)"(reference=w1086) -> ("Label.Text"=w1084:string)  [unwired: 1 in, 2 out]
            n80 = case shown="\"XY Correction Active\"" w1084 {
              tunnel: w1083 -> [_ w1091 w1094 w1097]
              tunnel: w1082 -> [w1089 w1092 w1095 w1098]
              tunnel: [w1089 w1090 w1093 w1096] -> w1081
              frame Default {
              }
              frame "XY Correction Active" {
                n81 = Bundle By Name(cluster=w1092, "XY Correction Active"=w1091) -> (w1090:T8)
              }
              frame "Z Correction Active" {
                n82 = Bundle By Name(cluster=w1095, "Z Correction Active"=w1094) -> (w1093:T8)
              }
              frame "Abort If Error" {
                n83 = Bundle By Name(cluster=w1098, "Abort If Error"=w1097) -> (w1096:T8)
              }
            }
            n84 = Bundle By Name(cluster=w1081, "Actions"=4Pi_Obj_Lock_-_Actions."Idle") -> (w1079:T8)
            n85 = Send Notification(notification=w1079, notifier=w1085) -> ()  [unwired: 1 in, 2 out]
          }
          event "Z Drift Threshold", "Z Stage Move Limit (µm)", "XY Drift Threshold", "XY Stage Move Limit (µm)", "P (Proportional)", "I (Integral)", "D (Derivative)", "Sample Z Step Size (µm)": Value Change {
            n86 = event-data() -> ("NewVal"=w1103:dbl, "CtlRef"=w1104:refnum<vi>)  [unwired: 1 in]
            n87 = Get Notifier Status(notifier=w1105) -> (notifier out=w1102:refnum<notifier>, current notification=w1106:T8)  [unwired: 1 in, 3 out]
            n88 = property class="DigNum (strict)"(reference=w1104) -> ("Label.Text"=w1107:string)  [unwired: 1 in, 2 out]
            n89 = case shown="\"Sample Z Step Size (µm)\"" w1107 {
              tunnel: w1103 -> [_ w1111 w1114 w1117 w1120 w1125 w1131 w1137 w1141]
              tunnel: w1106 -> [w1109 w1112 w1115 w1118 w1121 w1124 w1130 w1136 w1142]
              tunnel: [w1109 w1110 w1113 w1116 w1119 w1122 w1128 w1134 w1140] -> w1100
              frame Default {
              }
              frame "Z Drift Threshold" {
                n90 = Bundle By Name(cluster=w1112, "Z Drift Threshold"=w1111) -> (w1110:T8)
              }
              frame "Z Stage Move Limit (µm)" {
                n91 = Bundle By Name(cluster=w1115, "Z Stage Move Limit (µm)"=w1114) -> (w1113:T8)
              }
              frame "XY Drift Threshold" {
                n92 = Bundle By Name(cluster=w1118, "XY Drift Threshold"=w1117) -> (w1116:T8)
              }
              frame "XY Stage Move Limit (µm)" {
                n93 = Bundle By Name(cluster=w1121, "XY Stage Move Limit (µm)"=w1120) -> (w1119:T8)
              }
              frame "P (Proportional)" {
                n94 = Unbundle By Name(w1124) -> ("PID Values"=w1127:dbl[])
                n95 = Replace Array Subset(array=w1127, new element=w1125, index=0) -> (w1123:dbl[])
                n96 = Bundle By Name(cluster=w1124, "PID Values"=w1123) -> (w1122:T8)
              }
              frame "I (Integral)" {
                n97 = Unbundle By Name(w1130) -> ("PID Values"=w1133:dbl[])
                n98 = Replace Array Subset(array=w1133, new element=w1131, index=1) -> (w1129:dbl[])
                n99 = Bundle By Name(cluster=w1130, "PID Values"=w1129) -> (w1128:T8)
              }
              frame "D (Derivative)" {
                n100 = Unbundle By Name(w1136) -> ("PID Values"=w1139:dbl[])
                n101 = Replace Array Subset(array=w1139, new element=w1137, index=2) -> (w1135:dbl[])
                n102 = Bundle By Name(cluster=w1136, "PID Values"=w1135) -> (w1134:T8)
              }
              frame "Sample Z Step Size (µm)" {
                n103 = Bundle By Name(cluster=w1142, "Z Step Size (µm)"=w1141) -> (w1140:T8)
              }
            }
            n104 = Bundle By Name(cluster=w1100, "Actions"=4Pi_Obj_Lock_-_Actions."Idle") -> (w1099:T8)
            n105 = Send Notification(notification=w1099, notifier=w1102) -> ()  [unwired: 1 in, 2 out]
          }
          event "Sample Z Step No.": Value Change {
            n106 = event-data() -> ("NewVal"=w1144:u32)  [unwired: 1 in]
            n107 = for {
              N: w1144 -> [_]
              tunnel: [w1163] -> w1148 mode=indexing
              tunnel: [w1152] -> w1147 mode=indexing
              i -> [w1162]
              w1153 = T12 3 items=["Grayscale (U8)", "Grayscale (I16)", "Grayscale (SGL)", "Complex (CSG)", "RGB (U32)", "HSL (U32)", "RGB (U64)", "Grayscale (U16)"] ("Image Type")
              w1158 = T12 2 items=["Grayscale (U8)", "Grayscale (I16)", "Grayscale (SGL)", "Complex (CSG)", "RGB (U32)", "HSL (U32)", "RGB (U64)", "Grayscale (U16)"] ("Image Type")
              w1154 = 10 ("Border Size")
              n108 = Number To Decimal String(number=w1162, width (-)=i16 1) -> (decimal integer string=w1160:string)
              n109 = Concatenate Strings("Ref Stack " ("string"), w1160) -> (w1156:string)
              n110 = call "IMAQ Create"("Border Size"=w1154, "Image Name"=w1156, "Image Type"=w1158) -> ("New Image"=w1163:T9)  [unwired: 2 in, 1 out]
              n111 = Concatenate Strings("FFT" ("string"), w1156) -> (w1155:string)
              n112 = call "IMAQ Create"("Border Size"=w1154, "Image Name"=w1155, "Image Type"=w1153) -> ("New Image"=w1152:T9)  [unwired: 2 in, 1 out]
            }
            n113 = Get Notifier Status(notifier=w1146) -> (notifier out=w1150:refnum<notifier>, current notification=w1151:T8)  [unwired: 1 in, 3 out]
            n114 = Bundle By Name(cluster=w1151, "Actions"=4Pi_Obj_Lock_-_Actions."Idle", "Z Step No."=w1144, "Ref Stack (SGL)"=w1148, "Ref FFT Stack (CSG)"=w1147) -> (w1149:T8)
            n115 = Send Notification(notification=w1149, notifier=w1150) -> ()  [unwired: 1 in, 2 out]
          }
          event "Frame Accumulations": Value Change {
            n116 = event-data() -> ("NewVal"=w1166:u16)  [unwired: 1 in]
            n117 = Get Notifier Status(notifier=w1169) -> (notifier out=w1168:refnum<notifier>, current notification=w1167:T8)  [unwired: 1 in, 3 out]
            n118 = Bundle By Name(cluster=w1167, "Actions"=4Pi_Obj_Lock_-_Actions."Idle", "Frame Accumulations"=w1166) -> (w1165:T8)
            n119 = Send Notification(notification=w1165, notifier=w1168) -> ()  [unwired: 1 in, 2 out]
          }
          event "Update Delay (ms)": Value Change {
            n120 = event-data() -> ("NewVal"=w1173:i32)  [unwired: 1 in]
            n121 = Get Notifier Status(notifier=w1176) -> (notifier out=w1175:refnum<notifier>, current notification=w1174:T8)  [unwired: 1 in, 3 out]
            n122 = Bundle By Name(cluster=w1174, "Actions"=4Pi_Obj_Lock_-_Actions."Idle", "Update Delay (ms)"=w1173) -> (w1172:T8)
            n123 = Send Notification(notification=w1172, notifier=w1175) -> ()  [unwired: 1 in, 2 out]
          }
          event "Save Lock Settings": Value Change {
            n124 = event-data() -> ()  [unwired: 1 in, 1 out]
            n125 = Wait on Notification(notifier=w1205) -> (notification=w1203:T8)  [unwired: 3 in, 3 out]
            n126 = Unbundle By Name(w1203) -> ("Z Step Size (µm)"=w1179:dbl, "Z Step No."=w1178:u32, "Z Drift Threshold"=w1202:dbl, "Z Stage Move Limit (µm)"=w1201:dbl, "XY Drift Threshold"=w1200:dbl, "XY Stage Move Limit (µm)"=w1199:dbl, "Frame Accumulations"=w1198:u16, "Abort If Error"=w1197:bool, "Z Correction Active"=w1196:bool, "XY Correction Active"=w1195:bool, "PID Values"=w1185:dbl[])
            n127 = local read "Invert X Axis"() -> (w1183:bool)
            n128 = local read "Invert Y Axis"() -> (w1182:bool)
            n129 = local read "Invert Z Axis"() -> (w1181:bool)
            n130 = local read "Flip XY Axis"() -> (w1184:bool)
            n131 = Bundle By Name(cluster=T7 {"Z Drift Threshold"=0.05, "Z Stage Move Limit (µm)"=1.0, "XY Drift Threshold"=0.05, "XY Stage Move Limit (µm)"=1.0, "Frame Accumulations"=10, "Abort If Error"=FALSE, "Flip XY Axis"=FALSE, "Invert X Axis"=FALSE, "Invert Y Axis"=FALSE, "Invert Z Axis"=FALSE, "Z Correction Active"=TRUE, "XY Correction Active"=TRUE, "PID Values"=[], "Update Delay (ms)"=0, "Sample Z Step Size (µm)"=2.0, "Sample Z Step No."=2, "Z Update Scale Factor"=2.0, "Y Update Scale Factor"=2.0, "X Update Scale Factor"=2.0} ("Lock Settings"), "Sample Z Step Size (µm)"=w1179, "Sample Z Step No."=w1178, "Z Drift Threshold"=w1202, "Z Stage Move Limit (µm)"=w1201, "XY Drift Threshold"=w1200, "XY Stage Move Limit (µm)"=w1199, "Frame Accumulations"=w1198, "Abort If Error"=w1197, "Z Correction Active"=w1196, "XY Correction Active"=w1195, "PID Values"=w1185, "Flip XY Axis"=w1184, "Invert X Axis"=w1183, "Invert Y Axis"=w1182, "Invert Z Axis"=w1181) -> (w1194:T7)
            n132 = control-ref of="This VI"() -> (w1192:refnum<vi>)
            n133 = Flatten To JSON(anything=w1194) -> (JSON string=w1187:string)  [unwired: 2 in, 1 out]
            n134 = property class="VI"(reference=w1192) -> ("Path"=w1189:path)  [unwired: 1 in, 2 out]
            n135 = Strip Path(path=w1189) -> (stripped path=w1188:path)  [unwired: 1 out]
            n136 = Build Path(base path=w1188, name or relative path="4Pi Objective Lock Default Settings") -> (appended path=w1190:path)
            n137 = Build Path(base path=w1190, name or relative path="Default Obj Lock Settings.json") -> (appended path=w1186:path)
            n138 = Write to Text File(file (use dialog)=w1186, text=w1187) -> (refnum out=w1180:refnum<file>)  [unwired: 2 in, 2 out]
            n139 = Close File(refnum=w1180) -> ()  [unwired: 1 in, 2 out]
          }
          event "Start Lock": Value Change {
            n140 = event-data() -> ("NewVal"=w1212:bool)  [unwired: 1 in]
            n141 = Select(t=4Pi_Obj_Lock_-_Actions."Start Lock", s=w1212, f=4Pi_Obj_Lock_-_Actions."Abort" ("Actions")) -> (s? t:f=w1210:T6)
            n142 = Get Notifier Status(notifier=w1215) -> (notifier out=w1214:refnum<notifier>, current notification=w1213:T8)  [unwired: 1 in, 3 out]
            n143 = Bundle By Name(cluster=w1213, "Actions"=w1210, "Running?"=TRUE) -> (w1209:T8)
            n144 = Send Notification(notification=w1209, notifier=w1214) -> ()  [unwired: 1 in, 2 out]
          }
          event "Restart Lock": Value Change {
            n145 = event-data() -> ()  [unwired: 1 in, 1 out]
            n146 = Get Notifier Status(notifier=w1222) -> (notifier out=w1221:refnum<notifier>, current notification=w1220:T8)  [unwired: 1 in, 3 out]
            n147 = Bundle By Name(cluster=w1220, "Actions"=4Pi_Obj_Lock_-_Actions."Restart Lock" ("t")) -> (w1219:T8)
            n148 = local write "Start Lock"(TRUE ("Start Lock")) -> ()
            n149 = Send Notification(notification=w1219, notifier=w1221) -> ()  [unwired: 1 in, 2 out]
          }
          event "Quit": Value Change {
            # "Turn off the OBJ lock before quiting."
            n150 = event-data() -> ("NewVal"=w1233:bool)  [unwired: 1 in]
            n151 = Get Notifier Status(notifier=w1228) -> (notifier out=w1226:refnum<notifier>, current notification=w1224:T8)  [unwired: 1 in, 3 out]
            n152 = Unbundle By Name(w1224) -> ("Running?"=w1227:bool)
            n153 = case shown="True" w1227 {
              tunnel: w1226 -> [w1234 w1238]
              tunnel: [w1234 w1235] -> w1225
              tunnel: w1224 -> [_ w1240]
              frame False {
              }
              frame True {
                n154 = Bundle By Name(cluster=w1240, "Actions"=4Pi_Obj_Lock_-_Actions."Abort") -> (w1237:T8)
                n155 = Send Notification(notification=w1237, notifier=w1238) -> (notifier out=w1236:refnum<notifier>)  [unwired: 1 in, 1 out]
                n156 = while {
                  tunnel: w1236 -> [w1250]
                  tunnel: [w1245] -> w1235
                  i -> [w1244]
                  stop <- w1246 stop-if-true
                  n157 = Get Notifier Status(notifier=w1250) -> (notifier out=w1245:refnum<notifier>, # waiting=w1249:i32)  [unwired: 1 in, 3 out]
                  n158 = Greater?(x=w1244, y=1500) -> (0:w1242:bool)
                  n159 = Less?(x=w1249, y=1) -> (x < y?=w1247:bool)
                  n160 = Or(x=w1247, y=w1242) -> (x .or. y?=w1246:bool)
                  n161 = Wait (ms)(milliseconds to wait=u32 1) -> ()  [unwired: 1 out]
                }
              }
            }
            n162 = Get Notifier Status(notifier=w1225) -> (notifier out=w1230:refnum<notifier>, current notification=w1232:T8)  [unwired: 1 in, 3 out]
            n163 = Bundle By Name(cluster=w1232, "Actions"=4Pi_Obj_Lock_-_Actions."Quit") -> (w1229:T8)
            n164 = Send Notification(notification=w1229, notifier=w1230) -> ()  [unwired: 1 in, 2 out]
          }
        }
      }
      n165 = while {
        tunnel: w196 -> [w222]
        tunnel: w194 -> [w210]
        tunnel: w193 -> [w209]
        tunnel: w195 -> [w221]
        stop <- w217 stop-if-true
        # "Column 1 - Target Lock Values\nColumn 2 - Current Values\nColumn 3 - Differnce Values\nColumn 4 - Initial XYZ Stage Positions"
        n166 = Wait on Notification(notifier=w221, ignore previous (F)=FALSE) -> (notifier out=w216:refnum<notifier>, notification=w219:T8)  [unwired: 2 in, 2 out]
        n167 = Unbundle By Name(w219) -> ("Actions"=w211:T6)
        n168 = Equal?(x=4Pi_Obj_Lock_-_Actions."Quit", y=w211) -> (x = y?=w217:bool)
        n169 = Initialize Array(0.0 ("element"), 3 ("dimension size"), 4 ("dimension size")) -> (w213:dbl[][])
        n170 = while {
          shift-right: [w229] -> _
          shift-left: w211 -> [w237]
          tunnel: w222 -> [w241]
          tunnel: w210 -> [w240]
          tunnel: w209 -> [w239]
          tunnel: w216 -> [w235]
          shift-right: [w223] -> _
          shift-left: w213 -> [w224]
          stop <- w236 stop-if-true
          w231 = 4Pi_Obj_Lock_-_Actions."Abort" ("x")
          n171 = case shown="\"Check Drift cc\"" w237 {
            selector: w237 -> [_ _ _ _ _ _ _ _ _ _ _ _ _ w793 _ _ _ _ _ _]
            tunnel: w241 -> [_ w262 _ w366 _ _ w477 w511 w555 _ w621 _ _ _ _ _ _ w1032 _ _]
            tunnel: w240 -> [_ w295 _ _ _ _ w453 _ _ _ _ _ w717 w797 _ _ _ _ _ _]
            tunnel: w239 -> [_ w294 w323 w367 _ w427 w452 _ _ _ _ _ w716 _ w875 _ _ _ _ _]
            tunnel: FALSE -> [w244 w307 w319 w365 w405 w423 w480 w542 w557 w594 w651 w699 w723 w823 w880 w1007 w1019 w1036 _ _]
            tunnel: [4Pi_Obj_Lock_-_Actions."Exit Loop" ("x") w264 4Pi_Obj_Lock_-_Actions."Get Ref Stack" ("x") w370 4Pi_Obj_Lock_-_Actions."Move To Init Z" ("x") 4Pi_Obj_Lock_-_Actions."Get Initial Position" ("x") w472 w525 w560 4Pi_Obj_Lock_-_Actions."Get Current Position" ("x") w638 w677 w727 w812 w856 4Pi_Obj_Lock_-_Actions."Delay" ("x") 4Pi_Obj_Lock_-_Actions."Get Current Z Position" ("x") 4Pi_Obj_Lock_-_Actions."Exit Loop" ("x") 4Pi_Obj_Lock_-_Actions."Exit Loop" ("x") 4Pi_Obj_Lock_-_Actions."Quit" ("x")] -> w230
            tunnel: [w244 w307 w319 w365 w405 w423 w480 w542 w557 w594 w651 w699 w723 w823 w880 w1007 w1019 w1036 TRUE TRUE] -> w236
            tunnel: w235 -> [w243 w278 w324 w369 w410 w421 w479 w541 w567 w616 w650 w698 w758 w822 w878 w1005 w1017 w1040 w1046 w1050]
            tunnel: [w243 w273 w322 w368 w407 w421 w479 w533 w566 w592 w649 w697 w726 w821 w877 w1004 w1013 w1039 w1046 w1049] -> w234
            tunnel: w224 -> [w242 w291 w318 w364 w404 w422 w465 w540 w556 w593 w626 w687 w722 w783 w854 w986 w1016 w1035 w1045 w1058]
            tunnel: [w242 w290 w318 w364 w404 w422 w464 w539 w556 w593 w625 w684 w722 w783 w854 w986 w1016 w1035 w1045 w1058] -> w223
            frame "Idle", Default {
            }
            frame "Start Lock" {
              w247 = T17 [] ("History Data")
              w287 = FALSE ("Move Limit Error")
              w292 = Stage_Actions."Get Position" ("Actions")
              n172 = control-ref of="This VI"() -> (w305:refnum<vi>)
              n173 = call "Stages Messenger.vi"("Stage Notifier Name"=w295, "Actions"=w292) -> ("Positions"=w296:dbl[])  [unwired: 9 in, 4 out]
              n174 = call "Stages Messenger.vi"("Stage Notifier Name"=w294, "Actions"=w292) -> ("Positions"=w297:dbl[])  [unwired: 9 in, 4 out]
              n175 = property class="VI"(reference=w305) -> ("Path"=w302:path)  [unwired: 1 in, 2 out]
              n176 = local write "Move Limit Error"(w287) -> ()
              n177 = local write "Fit Error"(w287) -> ()
              n178 = Index Array(array=w297, index=0) -> (element=w293:dbl)
              n179 = Strip Path(path=w302) -> (stripped path=w301:path)  [unwired: 1 out]
              n180 = Build Path(base path=w301, name or relative path="4Pi Objective Lock Default Settings") -> (appended path=w303:path)
              n181 = Build Array (concatenate)(w296, w293) -> (w272:dbl[])
              n182 = Build Path(base path=w303, name or relative path="Initial Stage Positions.json") -> (appended path=w299:path)
              n183 = Flatten To JSON(anything=w272) -> (JSON string=w300:string)  [unwired: 2 in, 1 out]
              n184 = Replace Array Subset(array=w291, new element=w272, index (col)=3 ("disabled index (col)")) -> (w290:dbl[][])  [unwired: 1 in]
              n185 = Index Array(array=w272, index #1=0 ("index"), index #2=1 ("index"), index #3=2 ("index")) -> (element #1=w268:dbl, element #2=w266:dbl, element #3=w267:dbl)
              n186 = Write to Text File(file (use dialog)=w299, text=w300) -> (refnum out=w288:refnum<file>)  [unwired: 2 in, 2 out]
              n187 = local write "X Axis Position (µm)"(w268) -> ()
              n188 = local write "Y Axis Position (µm)"(w266) -> ()
              n189 = local write "Z Axis Position (µm)"(w267) -> ()
              n190 = Get Notifier Status(notifier=w278) -> (notifier out=w273:refnum<notifier>, current notification=w277:T8)  [unwired: 1 in, 3 out]
              n191 = Close File(refnum=w288) -> ()  [unwired: 1 in, 2 out]
              n192 = Unbundle By Name(w277) -> ("Cur Image (SGL)"=w276:T9)
              n193 = Unbundle By Name(w277) -> ("Z Step No."=w275:u32, "Ref Stack (SGL)"=w274:T9[])
              n194 = call "Camera Messenger.vi"("Notifier Name"=w262, "General Camera Actions"=Generic_Camera_Actions."Get ROI", "Camera ROI"=T14 {"H_Offset"=0, "V_Offset"=0, "H_Width"=0, "V_Width"=0} ("General Camera ROI")) -> ("Notifier Name Dup"=w259:string, "Camera ROI"=w279:T14)  [unwired: 7 in, 4 out]
              n195 = Unbundle By Name(w279) -> ("H_Width"=w284:u16, "V_Width"=w282:u16)
              n196 = To Long Integer(number=w284) -> (32bit integer=w283:i32)
              n197 = To Long Integer(number=w282) -> (32bit integer=w281:i32)
              n198 = Initialize Array(sgl 0.0 ("element"), w283, w281) -> (w248:sgl[][])
              n199 = for {
                N: w275 -> [_]
                tunnel: w248 -> [w316]
                tunnel: w274 -> [w317] mode=indexing
                n200 = call "IMAQ ArrayToImage"("Image Pixels (Float)"=w316, "Image"=w317) -> ()  [unwired: 8 in, 2 out]
              }
              n201 = call "IMAQ ArrayToImage"("Image Pixels (Float)"=w248, "Image"=w276) -> ()  [unwired: 8 in, 2 out]
              n202 = Array Size(array=w248) -> (size(s)=w254:i32[])
              n203 = To Double Precision Float(number=w254) -> (double precision float=w257:dbl[])
              n204 = call "Camera Messenger.vi"("Notifier Name"=w259, "General Camera Actions"=Generic_Camera_Actions."Live Preview") -> ("Notifier Name Dup"=w260:string)  [unwired: 8 in, 5 out]
              n205 = Divide(x=w257, y=2.0 ("index")) -> (x/y=w255:dbl[])
              n206 = while {
                tunnel: w260 -> [w314]
                tunnel: [w309] -> w258
                i -> [w313]
                stop <- w310 stop-if-true
                n207 = call "Camera Messenger.vi"("Notifier Name"=w314, "General Camera Actions"=Generic_Camera_Actions."Status") -> ("Running?"=w311:bool)  [unwired: 8 in, 5 out]
                n208 = Greater?(x=w313, y=3000) -> (0:w309:bool)
                n209 = Or(x=w311, y=w309) -> (x .or. y?=w310:bool)
                n210 = Wait (ms)(milliseconds to wait=u32 1) -> ()  [unwired: 1 out]
              }
              n211 = Round Toward -Infinity(1:w255) -> (0:w253:dbl[])
              n212 = Index Array(array=w253, index #1=0 ("index"), index #2=1 ("index")) -> (element #1=→"Target Y Position cc (px)":dbl, element #2=→"Target X Position cc (px)":dbl)
              n213 = Select(t=4Pi_Obj_Lock_-_Actions."Exit Loop", s=w258, f=4Pi_Obj_Lock_-_Actions."Get Target Z Position" ("x")) -> (s? t:f=w264:T6)
              n214 = property on="X Target and Fit Position (µm)" class="WFChart (strict)"("History Data"=w247) -> ()  [unwired: 2 in, 2 out]
              n215 = property on="Y Target and Fit Position (µm)" class="WFChart (strict)"("History Data"=w247) -> ()  [unwired: 2 in, 2 out]
              n216 = property on="Z Target and Fit Value (µm)" class="WFChart (strict)"("History Data"=w247) -> ()  [unwired: 2 in, 2 out]
              n217 = property on="CC Max" class="WFChart (strict)"("History Data"=cluster{"pixel size (µm)":dbl}[] []) -> ()  [unwired: 2 in, 2 out]
            }
            frame "Get Target Z Position" {
              w345 = 0.0 ("Target Z (µm)")
              n218 = Get Notifier Status(notifier=w324) -> (notifier out=w343:refnum<notifier>, current notification=w348:T8)  [unwired: 1 in, 3 out]
              n219 = Unbundle By Name(w348) -> ("Z Step No."=w341:u32, "Z Step Size (µm)"=w340:dbl, "Z Stage Move Limit (µm)"=w338:dbl)
              n220 = Unbundle By Name(w348) -> ("Z Step No."=w333:u32, "Z Step Size (µm)"=w346:dbl)
              n221 = Divide(x=w341, y=2.0) -> (x/y=w331:dbl)
              n222 = Round Toward -Infinity(1:w331) -> (0:w330:dbl)
              n223 = Multiply(x=w330, y=w340) -> (x*y=w335:dbl)
              n224 = Decrement(x=w333) -> (x-1=w332:u32)
              n225 = Negate(x=w335) -> (-x=w334:dbl)
              n226 = Negate(x=w338) -> (-x=w339:dbl)
              n227 = In Range and Coerce(upper limit=w338, x=w334, lower limit=w339) -> (coerced(x)=w336:dbl)  [unwired: 1 out]
              n228 = Add(x=w345, y=w336) -> (x+y=w337:dbl)
              n229 = Build Array(w337) -> (w347:dbl[])
              n230 = for {
                N: w332 -> [_]
                tunnel: w346 -> [w359]
                shift-right: [w360] -> w344
                shift-left: w347 -> [w361]
                shift-right: [w357] -> _
                shift-left: w337 -> [w358]
                n231 = Add(x=w358, y=w359) -> (x+y=w357:dbl)
                n232 = Build Array (concatenate)(w361, w357) -> (w360:dbl[])
              }
              n233 = Build Array(w336) -> (w349:dbl[])
              n234 = call "Stages Messenger.vi"("Stage Notifier Name"=w323, "Actions"=Stage_Actions."MVR", "Setpoint"=w349, "Axis"=bool[] [TRUE], "Exit While Busy?"=FALSE) -> ("Stage Notifier Name (Dup)"=w328:string, "Status"=w329:T18)  [unwired: 6 in, 3 out]
              n235 = case shown="Default" w329 {
                tunnel: [w355] -> w327
                tunnel: w328 -> [w355]
                frame Default {
                  n236 = Wait (ms)(milliseconds to wait=u32 150) -> ()  [unwired: 1 out]
                }
              }
              n237 = Bundle By Name(cluster=w348, "Sample Z (µm)"=w344) -> (w342:T8)
              n238 = call "Stages Messenger.vi"("Stage Notifier Name"=w327, "Actions"=Stage_Actions."Get Position") -> ("Positions"=w325:dbl[])  [unwired: 9 in, 4 out]
              n239 = Index Array(array=w325, index=0) -> (element=w320:dbl)
              n240 = Send Notification(notification=w342, notifier=w343) -> (notifier out=w322:refnum<notifier>)  [unwired: 1 in, 1 out]
              n241 = local write "Z Axis Position (µm)"(w320) -> ()
              "Target Z (µm)" <- w345
            }
            frame "Get Ref Stack" {
              n242 = Get Notifier Status(notifier=w369) -> (notifier out=w368:refnum<notifier>, current notification=w363:T8)  [unwired: 1 in, 3 out]
              n243 = Unbundle By Name(w363) -> ("Z Step No."=w373:u32, "Ref Stack (SGL)"=w372:T9[])
              n244 = Unbundle By Name(w363) -> ("Frame Accumulations"=w362:u16)
              n245 = Unbundle By Name(w363) -> ("Z Step Size (µm)"=w371:dbl)
              n246 = while {
                tunnel: w366 -> [w391]
                tunnel: w373 -> [w388]
                tunnel: w368 -> [w390]
                tunnel: [w380] -> w370
                tunnel: w372 -> [w379] mode=indexing
                tunnel: w371 -> [w378]
                tunnel: w367 -> [w377]
                tunnel: w362 -> [w374]
                i -> [w387]
                stop <- w383 stop-if-true
                n247 = flat-sequence {
                  tunnel: w391 -> [w394]
                  tunnel: w379 -> [w392]
                  tunnel: w374 -> [w393]
                  tunnel: w378 -> [w398]
                  tunnel: w377 -> [w397]
                  frame #0 {
                    n248 = call "Generic Camera Get New Camera Image.vi"("Camera Notifier Name"=w394, "Frames"=w393) -> ("Image - U16"=w396:u16[][])  [unwired: 11 in, 2 out]
                    n249 = To Single Precision Float(number=w396) -> (single precision float=w395:sgl[][])
                    n250 = call "IMAQ ArrayToImage"("Image Pixels (Float)"=w395, "Image"=w392) -> ()  [unwired: 8 in, 2 out]
                  }
                  frame #1 {
                    n251 = Build Array(w398) -> (w402:dbl[])
                    n252 = call "Stages Messenger.vi"("Stage Notifier Name"=w397, "Actions"=Stage_Actions."MVR", "Setpoint"=w402, "Axis"=bool[] [TRUE], "Exit While Busy?"=FALSE) -> ()  [unwired: 6 in, 5 out]
                  }
                  frame #2 {
                    n253 = Wait (ms)(milliseconds to wait=u32 150) -> ()  [unwired: 1 out]
                  }
                }
                n254 = Get Notifier Status(notifier=w390) -> (current notification=w382:T8)  [unwired: 1 in, 4 out]
                n255 = To Unsigned Long Integer(number=w387) -> (unsigned 32bit integer=w386:u32)
                n256 = Increment(x=w386) -> (x+1=w389:u32)
                n257 = Unbundle By Name(w382) -> ("Running?"=w385:bool)
                n258 = Greater Or Equal?(x=w389, y=w388) -> (x >= y?=w384:bool)
                n259 = Not(x=w385) -> (.not. x?=w381:bool)
                n260 = Or(x=w381, y=w384) -> (x .or. y?=w383:bool)
                n261 = Select(t=4Pi_Obj_Lock_-_Actions."Abort" ("x"), s=w381, f=4Pi_Obj_Lock_-_Actions."Cal Ref FFT") -> (s? t:f=w380:T6)
              }
            }
            frame "Cal Ref FFT" {
              n262 = Get Notifier Status(notifier=w410) -> (notifier out=w407:refnum<notifier>, current notification=w411:T8)  [unwired: 1 in, 3 out]
              n263 = Unbundle By Name(w411) -> ("Ref Stack (SGL)"=w409:T9[], "Ref FFT Stack (CSG)"=w408:T9[])
              n264 = for {
                tunnel: w409 -> [w413] mode=indexing
                tunnel: w408 -> [w412] mode=indexing
                n265 = call "4Pi Obj Lock - Norm FFT.vi"("FFT Image Dst"=w412, "Image In"=w413) -> ()  [unwired: 8 in, 2 out]
              }
            }
            frame "Move To Init Z" {
              # "initial z stage position"
              n266 = Index Array(array=w422, index (row)=2, index (col)=3 ("disabled index (col)")) -> (element=w424:dbl)
              n267 = flat-sequence {
                tunnel: w427 -> [w437]
                tunnel: [w436] -> w429
                tunnel: w424 -> [w432]
                tunnel: [w430] -> w428
                tunnel: w429 -> [w441]
                tunnel: w428 -> [w440]
                tunnel: [w439] -> w414
                tunnel: [w446] -> w416
                tunnel: w414 -> [w446]
                frame #0 {
                  n268 = call "Stages Messenger.vi"("Stage Notifier Name"=w437, "Actions"=Stage_Actions."Get Position") -> ("Stage Notifier Name (Dup)"=w436:string, "Positions"=w434:dbl[])  [unwired: 9 in, 3 out]
                  n269 = Index Array(array=w434, index=0) -> (element=w433:dbl)
                  n270 = Subtract(x=w432, y=w433) -> (x-y=w431:dbl)
                  n271 = Build Array(w431) -> (w430:dbl[])
                }
                frame #1 {
                  n272 = call "Stages Messenger.vi"("Stage Notifier Name"=w441, "Actions"=Stage_Actions."MVR", "Setpoint"=w440, "Axis"=bool[] [TRUE], "Exit While Busy?"=FALSE) -> ("Stage Notifier Name (Dup)"=w439:string)  [unwired: 6 in, 4 out]
                }
                frame #2 {
                  n273 = Wait (ms)(milliseconds to wait=u32 150) -> ()  [unwired: 1 out]
                }
              }
              n274 = call "Stages Messenger.vi"("Stage Notifier Name"=w416, "Actions"=Stage_Actions."Get Position") -> ("Positions"=w418:dbl[])  [unwired: 9 in, 4 out]
              n275 = Index Array(array=w418, index=0) -> (element=w417:dbl)
              n276 = local write "Z Axis Position (µm)"(w417) -> ()
            }
            frame "Restart Lock" {
              w447 = T17 [] ("History Data")
              w448 = FALSE ("Move Limit Error")
              # "Make sure the camera is running, if not abort."
              n277 = control-ref of="This VI"() -> (w470:refnum<vi>)
              n278 = call "Camera Messenger.vi"("Notifier Name"=w477, "General Camera Actions"=Generic_Camera_Actions."Live Preview") -> ("Notifier Name Dup"=w476:string)  [unwired: 8 in, 5 out]
              n279 = property class="VI"(reference=w470) -> (error out=w456:errorcluster, "Path"=w467:path)  [unwired: 1 in, 1 out]
              n280 = while {
                tunnel: w476 -> [w506]
                tunnel: [w501] -> w475
                i -> [w505]
                stop <- w502 stop-if-true
                n281 = call "Camera Messenger.vi"("Notifier Name"=w506, "General Camera Actions"=Generic_Camera_Actions."Status") -> ("Running?"=w503:bool)  [unwired: 8 in, 5 out]
                n282 = Greater?(x=w505, y=3000) -> (0:w501:bool)
                n283 = Or(x=w503, y=w501) -> (x .or. y?=w502:bool)
                n284 = Wait (ms)(milliseconds to wait=u32 1) -> ()  [unwired: 1 out]
              }
              n285 = Strip Path(path=w467) -> (stripped path=w466:path)  [unwired: 1 out]
              n286 = Build Path(base path=w466, name or relative path="4Pi Objective Lock Default Settings") -> (appended path=w468:path)
              n287 = Build Path(base path=w468, name or relative path="Initial Stage Positions.json") -> (appended path=w462:path)
              n288 = Read from Text File(file (use dialog)=w462, error in=w456) -> (refnum out=w461:refnum<file>, text=w460:string, error out=w459:errorcluster)  [unwired: 2 in, 1 out]
              n289 = Close File(refnum=w461, error in=w459) -> (error out=w458:errorcluster)  [unwired: 1 out]
              n290 = local write "Move Limit Error"(w448) -> ()
              n291 = local write "Fit Error"(w448) -> ()
              n292 = Unflatten From JSON(JSON string=w460, type and defaults=dbl[] [], error in (no error)=w458) -> (value=w454:dbl[], error out=w455:errorcluster)  [unwired: 4 in]
              n293 = case shown="Error" w455 {
                tunnel: w454 -> [w482 _]
                tunnel: w453 -> [w489 w494]
                tunnel: w452 -> [w488 w493]
                tunnel: [w482 w492] -> w451
                tunnel: u32 150 ("milliseconds to wait") -> [w481 w491]
                tunnel: [w481 w491] -> w449
                frame No Error {
                  w490 = Stage_Actions."MOVE" ("Actions")
                  n294 = Split 1D Array(array=w482, index=2) -> (first subarray=w486:dbl[], second subarray=w485:dbl[])
                  n295 = call "Stages Messenger.vi"("Stage Notifier Name"=w489, "Actions"=w490, "Setpoint"=w486, "Axis"=bool[] [TRUE, TRUE]) -> ()  [unwired: 7 in, 5 out]
                  n296 = call "Stages Messenger.vi"("Stage Notifier Name"=w488, "Actions"=w490, "Setpoint"=w485, "Axis"=bool[] [TRUE]) -> ()  [unwired: 7 in, 5 out]
                }
                frame Error {
                  w495 = Stage_Actions."Get Position" ("Actions")
                  n297 = call "Stages Messenger.vi"("Stage Notifier Name"=w494, "Actions"=w495) -> ("Positions"=w497:dbl[])  [unwired: 9 in, 4 out]
                  n298 = call "Stages Messenger.vi"("Stage Notifier Name"=w493, "Actions"=w495) -> ("Positions"=w498:dbl[])  [unwired: 9 in, 4 out]
                  n299 = Index Array(array=w498, index=0) -> (element=w496:dbl)
                  n300 = Build Array (concatenate)(w497, w496) -> (w492:dbl[])
                }
              }
              n301 = Wait (ms)(milliseconds to wait=w449) -> ()  [unwired: 1 out]
              n302 = Replace Array Subset(array=w465, new element=w451, index (col)=3 ("disabled index (col)")) -> (w464:dbl[][])  [unwired: 1 in]
              n303 = property on="X Target and Fit Position (µm)" class="WFChart (strict)"("History Data"=w447) -> ()  [unwired: 2 in, 2 out]
              n304 = property on="Y Target and Fit Position (µm)" class="WFChart (strict)"("History Data"=w447) -> ()  [unwired: 2 in, 2 out]
              n305 = property on="Z Target and Fit Value (µm)" class="WFChart (strict)"("History Data"=w447) -> ()  [unwired: 2 in, 2 out]
              n306 = Select(t=4Pi_Obj_Lock_-_Actions."Exit Loop" ("x"), s=w475, f=4Pi_Obj_Lock_-_Actions."Get Initial Position" ("x")) -> (s? t:f=w472:T6)
            }
            frame "Get Initial Position" {
              w518 = 0 ("index")
              # "Set target values"
              n307 = Get Notifier Status(notifier=w541) -> (notifier out=w534:refnum<notifier>, current notification=w510:T8)  [unwired: 1 in, 3 out]
              n308 = Unbundle By Name(w510) -> ("Frame Accumulations"=w509:u16)
              n309 = Bundle By Name(cluster=w510, "Running?"=TRUE) -> (w531:T8)
              n310 = Send Notification(notification=w531, notifier=w534) -> (notifier out=w533:refnum<notifier>)  [unwired: 1 in, 1 out]
              n311 = call "Generic Camera Get New Camera Image.vi"("Camera Notifier Name"=w511, "Frames"=w509) -> ("Image - U16"=w508:u16[][])  [unwired: 11 in, 2 out]
              n312 = call "2D Gaussian - Fit Image U16.vi"("Image In (U16)"=w508) -> ("Best Fit Params"=w538:T19, "Error Out"=w524:errorcluster)  [unwired: 13 in]
              n313 = Unbundle By Name(w524) -> ("status"=w523:bool)
              n314 = Cluster To Array(cluster=w538) -> (array=w537:dbl[])
              n315 = local write "Fit Error"(w523) -> ()
              n316 = Array Subset(array=w537, index=1, length=4) -> (w530:dbl[])
              n317 = Index Array(array=w530, index #1=0 ("index"), index #2=1 ("index"), index #3=2 ("index"), index #4=3 ("index")) -> (element #1=w512:dbl, element #2=w513:dbl, element #3=w520:dbl, element #4=w519:dbl)
              "Target X Position (px)" <- w512
              "Target Y Position (px)" <- w513
              n318 = Divide(x=w520, y=w519) -> (x/y=w514:dbl)
              "Target sx/sy" <- w514
              n319 = Replace Array Subset(array=w540, new element #1=w512, index (row) #1=0 ("disabled index (row)"), index (col) #1=w518, new element #2=w513, index (row) #2=1 ("disabled index (row)"), index (col) #2=w518, new element #3=w514, index (row) #3=2 ("disabled index (row)"), index (col) #3=w518) -> (w539:dbl[][])
              n320 = Select(t=4Pi_Obj_Lock_-_Actions."Abort" ("x"), s=w523, f=4Pi_Obj_Lock_-_Actions."Get Current Z Position" ("x")) -> (s? t:f=w525:T6)
            }
            frame "Get Current Z Position" {
              n321 = Get Notifier Status(notifier=w567) -> (notifier out=w566:refnum<notifier>, current notification=w554:T8)  [unwired: 1 in, 3 out]
              n322 = Unbundle By Name(w554) -> ("CC Image (SGL)"=w545:T9, "CC Image Max (SGL)"=w544:T9)
              n323 = Unbundle By Name(w554) -> ("Ref FFT Stack (CSG)"=w573:T9[])
              n324 = Unbundle By Name(w554) -> ("Cur Image (SGL)"=w550:T9, "Tmp Image FFT (CSG)"=w563:T9[])
              n325 = Unbundle By Name(w554) -> ("Sample Z (µm)"=w575:dbl[])
              n326 = Unbundle By Name(w554) -> ("Frame Accumulations"=w553:u16)
              n327 = call "Generic Camera Get New Camera Image.vi"("Camera Notifier Name"=w555, "Frames"=w553) -> ("Image - U16"=w552:u16[][])  [unwired: 11 in, 2 out]
              n328 = Index Array(array=w563, index #1=0 ("index"), index #2=1 ("index"), index #3=2 ("index")) -> (element #1=w561:T9, element #2=w547:T9, element #3=w546:T9)
              n329 = To Single Precision Float(number=w552) -> (single precision float=w549:sgl[][])
              n330 = call "IMAQ ArrayToImage"("Image Pixels (Float)"=w549, "Image"=w550) -> ("Image Out"=w551:T9)  [unwired: 8 in, 1 out]
              n331 = call "4Pi Obj Lock - Norm FFT.vi"("FFT Image Dst"=w561, "Image In"=w551) -> ("FFT Image Out"=w571:T9)  [unwired: 8 in, 1 out]
              n332 = call "IMAQ ComplexConjugate"("Image Src"=w571) -> ("Image Dst Out"=w570:T9)  [unwired: 3 in, 1 out]
              n333 = for {
                tunnel: [w580] -> w576 mode=indexing
                tunnel: w570 -> [w586]
                tunnel: w573 -> [w585] mode=indexing
                shift-right: [w580] -> _
                shift-left: sgl 0.0 ("Max CC") -> [w581]
                tunnel: w547 -> [w584]
                tunnel: w546 -> [w583]
                tunnel: w545 -> [w579]
                tunnel: w544 -> [w577]
                n334 = call "4Pi Obj Lock - Get Cross Correlation.vi"("Ref FFT image"=w585, "Cur FFT Image"=w586, "FFT CC image"=w584, "iFFT image"=w583, "CC image"=w579) -> ("Max CC"=w580:sgl, "CC image Out"=w578:T9)  [unwired: 8 in, 1 out]
                n335 = Greater?(x=w580, y=w581) -> (0:w582:bool)
                n336 = case shown="True" w582 {
                  tunnel: w578 -> [_ w588]
                  tunnel: w577 -> [_ w587]
                  frame False {
                  }
                  frame True {
                    n337 = call "IMAQ Copy"("Image Dst"=w587, "Image Src"=w588) -> ()  [unwired: 4 in, 2 out]
                  }
                }
              }
              n338 = To Double Precision Float(number=w576) -> (double precision float=w572:dbl[])
              n339 = call "4Pi Obj Lock - Find Peak Position.vi"("Fit Size"=2, "y"=w572, "x"=w575) -> ("Peak value"=→"CC Max Value":dbl, "Coerced Peak Position"=w569:dbl)  [unwired: 6 in, 1 out]
              "Measured Z (µm)" <- w569
              n340 = Not A Number/Path/Refnum?(number/path/refnum=w569) -> (NaN/Path/Refnum?=w568:bool)
              n341 = Select(t=4Pi_Obj_Lock_-_Actions."Get Current Z Position" ("x"), s=w568, f=4Pi_Obj_Lock_-_Actions."Get Current XY Position") -> (s? t:f=w560:T6)
            }
            frame "Get Current XY Position" {
              w604 = 3 ("edge size")
              n342 = Get Notifier Status(notifier=w616) -> (notifier out=w592:refnum<notifier>, current notification=w615:T8)  [unwired: 1 in, 3 out]
              n343 = Unbundle By Name(w615) -> ("CC Image Max (SGL)"=w614:T9)
              n344 = call "IMAQ ImageToArray"("Image"=w614) -> ("Image Pixels (Float)"=w601:sgl[][])  [unwired: 3 in, 4 out]
              n345 = call "4Pi Obj Lock - FFT shift 2D.vi"("Input image"=w601) -> ("fft shifted image"=w600:sgl[][])  [unwired: 10 in]
              n346 = call "4Pi Obj Lock - Crop Imag at Max.vi"("edge size"=w604, "Input array"=w600) -> ("Y"=w610:i32, "X"=w611:i32, "subarray"=w613:sgl[][])  [unwired: 6 in, 1 out]
              n347 = To Double Precision Float(number=w613) -> (double precision float=w590:dbl[][])
              n348 = Build Array(w611, w610) -> (w609:i32[])
              n349 = call "2D Gaussian - Fit -init.vi"("Image In (DBL)"=w590, "width"=10.0) -> ("Best Fit Params"=w612:T19)  [unwired: 12 in, 1 out]
              n350 = To Double Precision Float(number=w609) -> (double precision float=w606:dbl[])
              n351 = Unbundle By Name(w612) -> ("X Position"=w608:dbl, "Y Position"=w607:dbl)
              n352 = Build Array(w608, w607) -> (w605:dbl[])
              n353 = To Double Precision Float(number=w604) -> (double precision float=w603:dbl)
              n354 = Subtract(x=w605, y=w603) -> (x-y=w602:dbl[])
              n355 = Add(x=w602, y=w606) -> (x+y=w597:dbl[])
              n356 = Index Array(array=w597, index #1=0 ("index"), index #2=1 ("index")) -> (element #1=→"Measured X Position cc (px)":dbl, element #2=→"Measured Y Position cc (px)":dbl)
            }
            frame "Get Current Position" {
              w630 = 1 ("index")
              # "retake current image"
              # "Update current values"
              n357 = Get Notifier Status(notifier=w650) -> (notifier out=w649:refnum<notifier>, current notification=w618:T8)  [unwired: 1 in, 3 out]
              n358 = Unbundle By Name(w618) -> ("Abort If Error"=w643:bool, "Cur Image (SGL)"=w620:T9)
              n359 = case shown="True" TRUE {
                tunnel: w621 -> [_ w660]
                tunnel: w620 -> [w654 w657]
                tunnel: w618 -> [_ w659]
                tunnel: [w652 w656] -> w617
                frame False {
                  n360 = call "IMAQ ImageToArray"("Image"=w654) -> ("Image Pixels (Float)"=w653:sgl[][])  [unwired: 3 in, 4 out]
                  n361 = To Unsigned Word Integer(number=w653) -> (unsigned 16bit integer=w652:u16[][])
                }
                frame True {
                  n362 = Unbundle By Name(w659) -> ("Frame Accumulations"=w658:u16)
                  n363 = call "Generic Camera Get New Camera Image.vi"("Camera Notifier Name"=w660, "Frames"=w658) -> ("Image - U16"=w656:u16[][])  [unwired: 11 in, 2 out]
                  n364 = To Single Precision Float(number=w656) -> (single precision float=w655:sgl[][])
                  n365 = call "IMAQ ArrayToImage"("Image Pixels (Float)"=w655, "Image"=w657) -> ()  [unwired: 8 in, 2 out]
                }
              }
              n366 = call "2D Gaussian - Fit Image U16.vi"("Image In (U16)"=w617) -> ("Best Fit Params"=w648:T19, "Error Out"=w644:errorcluster)  [unwired: 13 in]
              n367 = Unbundle By Name(w644) -> ("status"=w642:bool)
              "Fit Error" <- w642
              n368 = And(x=w643, y=w642) -> (x .and. y?=w641:bool)
              n369 = Cluster To Array(cluster=w648) -> (array=w647:dbl[])
              n370 = Array Subset(array=w647, index=1, length=4) -> (w631:dbl[])
              n371 = Index Array(array=w631, index #1=0 ("index"), index #2=1 ("index"), index #3=2 ("index"), index #4=3 ("index")) -> (element #1=w622:dbl, element #2=w623:dbl, element #3=w633:dbl, element #4=w632:dbl)
              "Measured X Position (px)" <- w622
              "Measured Y Position (px)" <- w623
              n372 = Divide(x=w633, y=w632) -> (x/y=w624:dbl)
              "Measured sx/sy" <- w624
              n373 = Select(t=4Pi_Obj_Lock_-_Actions."Abort" ("x"), s=w641, f=4Pi_Obj_Lock_-_Actions."Check Drift" ("x")) -> (s? t:f=w638:T6)
              n374 = Replace Array Subset(array=w626, new element #1=w622, index (row) #1=0 ("disabled index (row)"), index (col) #1=w630, new element #2=w623, index (row) #2=1 ("disabled index (row)"), index (col) #2=w630, new element #3=w624, index (row) #3=2 ("disabled index (row)"), index (col) #3=w630) -> (w625:dbl[][])
            }
            frame "Check Drift" {
              # "Update the PID difference between target values and current values"
              # "Check if Sigma X / Sigma Y is over the limit"
              # "Check if XY values are over the limit"
              n375 = Get Notifier Status(notifier=w698) -> (notifier out=w697:refnum<notifier>, current notification=w696:T8)  [unwired: 1 in, 3 out]
              n376 = Unbundle By Name(w696) -> ("Z Correction Active"=w673:bool, "XY Correction Active"=w675:bool, "XY Drift Threshold"=w667:dbl, "Z Drift Threshold"=w663:dbl, "PID Values"=w695:dbl[])
              n377 = Index Array(array=w687, index (col) #1=0 ("disabled index (col)"), index (col) #2=1 ("index (col)")) -> (element #1=w689:dbl[], element #2=w688:dbl[])  [unwired: 2 in]
              n378 = local read "Metric scale sx/sy"() -> (w661:dbl)
              n379 = Array To Cluster(array=w695) -> (cluster=w669:T20)
              n380 = local read "pixel size (µm)"() -> (w666:dbl)
              n381 = Build Array(w669) -> (w694:T21)
              n382 = Divide(x=w667, y=w666) -> (x/y=w668:dbl)
              n383 = Divide(x=w663, y=w661) -> (x/y=w662:dbl)
              n384 = call-poly <vilib>:"PID.vi"("PID gains"=w694, "process variable"=w688, "setpoint"=w689) -> ("dt out (s)"=w664:dbl, "output"=w685:dbl[])  [unwired: 7 in]
              n385 = Build Array(w668, w668, w662) -> (w692:dbl[])
              n386 = local write "dt z (s)"(w664) -> ()
              n387 = Replace Array Subset(array=w687, new element=w685, index (col)=2 ("disabled index (col)")) -> (w684:dbl[][])  [unwired: 1 in]
              n388 = Absolute Value(x=w685) -> (abs(x)=w693:dbl[])
              n389 = Greater?(x=w693, y=w692) -> (0:w683:bool[])
              n390 = Split 1D Array(array=w683, index=2) -> (first subarray=w681:bool[], second subarray=w680:bool[])
              n391 = Or Array Elements(Boolean array=w681) -> (logical OR=w676:bool)
              n392 = Or Array Elements(Boolean array=w680) -> (logical OR=w665:bool)
              n393 = And(x=w675, y=w676) -> (x .and. y?=w674:bool)
              n394 = And(x=w673, y=w665) -> (x .and. y?=w672:bool)
              n395 = Build Array(w674, w672) -> (w679:bool[])
              n396 = Boolean Array To Number(Boolean array=w679) -> (number=w678:u32)
              n397 = case shown="3" w678 {
                tunnel: [4Pi_Obj_Lock_-_Actions."Update Plots" ("x") 4Pi_Obj_Lock_-_Actions."Move XY" ("x") 4Pi_Obj_Lock_-_Actions."Move Z" ("x") 4Pi_Obj_Lock_-_Actions."Move XYZ" ("x")] -> w677
                tunnel: [w700 TRUE FALSE w708] -> w671
                tunnel: [w700 FALSE TRUE w708] -> w670
                frame 0, Default {
                  w700 = FALSE
                  # "XYZ within limits, no move"
                }
                frame 1 {
                  # "X or Y outside limit, move XY"
                }
                frame 2 {
                  # "Sigma X / Y outside limit, move Z"
                }
                frame 3 {
                  w708 = TRUE
                  # "XYZ outside limit, move all"
                }
              }
              "XY Move" <- w671
              "Z Move" <- w670
            }
            frame "Check Drift cc" {
              w718 = Stage_Actions."Get Position" ("Actions")
              n398 = Get Notifier Status(notifier=w758) -> (notifier out=w726:refnum<notifier>, current notification=w744:T8)  [unwired: 1 in, 3 out]
              n399 = call "Stages Messenger.vi"("Stage Notifier Name"=w717, "Actions"=w718) -> ("Positions"=w715:dbl[])  [unwired: 9 in, 4 out]
              n400 = call "Stages Messenger.vi"("Stage Notifier Name"=w716, "Actions"=w718) -> ("Positions"=w719:dbl[])  [unwired: 9 in, 4 out]
              n401 = Index Array(array=w715, index #1=0 ("index"), index #2=1 ("index")) -> (element #1=w710:dbl, element #2=w711:dbl)
              n402 = Index Array(array=w719, index=0) -> (element=w712:dbl)
              n403 = local write "Z Axis Position (µm)"(w712) -> ()
              n404 = local write "Y Axis Position (µm)"(w711) -> ()
              n405 = local write "X Axis Position (µm)"(w710) -> ()
              n406 = Unbundle By Name(w744) -> ("XY Correction Active"=w734:bool, "XY Drift Threshold"=w761:dbl, "PID Values"=w759:dbl[])
              n407 = local read "Measured Y Position cc (px)"() -> (w755:dbl)
              n408 = local read "Measured X Position cc (px)"() -> (w756:dbl)
              n409 = Unbundle By Name(w744) -> ("Z Correction Active"=w735:bool, "Z Drift Threshold"=w737:dbl, "PID Values"=w743:dbl[])
              n410 = local read "Target X Position cc (px)"() -> (w754:dbl)
              n411 = local read "Target Y Position cc (px)"() -> (w753:dbl)
              n412 = Array To Cluster(array=w759) -> (cluster=w760:T20)
              n413 = local read "pixel size (µm)"() -> (w762:dbl)
              n414 = Array To Cluster(array=w743) -> (cluster=w742:T20)
              n415 = Build Array(w760) -> (w757:T21)
              n416 = Build Array(w754, w753) -> (w751:dbl[])
              n417 = Build Array(w756, w755) -> (w752:dbl[])
              n418 = local read "Measured Z (µm)"() -> (w739:dbl)
              n419 = local read "Target Z (µm)"() -> (w740:dbl)
              n420 = Divide(x=w761, y=w762) -> (x/y=w749:dbl)
              n421 = Subtract(x=w752, y=w751) -> (x-y=w750:dbl[])
              n422 = call-poly <vilib>:"PID.vi"("PID gains"=w757, "process variable"=w752, "setpoint"=w751) -> ("output"=→"dxy (px)":dbl[])  [unwired: 7 in, 1 out]
              n423 = Build Array(w749, w749) -> (w748:dbl[])
              n424 = Absolute Value(x=w750) -> (abs(x)=w747:dbl[])
              n425 = Subtract(x=w739, y=w740) -> (x-y=w741:dbl)
              n426 = call-poly <vilib>:"PID.vi"("PID gains"=w742, "process variable"=w739, "setpoint"=w740) -> ("dt out (s)"=→"dt z (s)":dbl, "output"=→"dz (µm)":dbl)  [unwired: 7 in]
              n427 = Greater?(x=w747, y=w748) -> (0:w746:bool[])
              n428 = Absolute Value(x=w741) -> (abs(x)=w738:dbl)
              n429 = Or Array Elements(Boolean array=w746) -> (logical OR=w745:bool)
              n430 = Greater?(x=w738, y=w737) -> (0:w736:bool)
              n431 = And(x=w734, y=w745) -> (x .and. y?=w729:bool)
              n432 = And(x=w735, y=w736) -> (x .and. y?=w728:bool)
              n433 = Build Array(w729, w728) -> (w730:bool[])
              n434 = Boolean Array To Number(Boolean array=w730) -> (number=w731:u32)
              n435 = case shown="2" w731 {
                tunnel: [4Pi_Obj_Lock_-_Actions."Update Plots" ("x") 4Pi_Obj_Lock_-_Actions."Move XY" ("x") 4Pi_Obj_Lock_-_Actions."Move Z" ("x") 4Pi_Obj_Lock_-_Actions."Move XYZ" ("x")] -> w727
                tunnel: [w763 TRUE FALSE w771] -> w725
                tunnel: [w763 FALSE TRUE w771] -> w724
                frame 0, Default {
                  w763 = FALSE
                  # "XYZ within limits, no move"
                }
                frame 1 {
                  # "X or Y outside limit, move XY"
                }
                frame 2 {
                  # "Sigma X / Y outside limit, move Z"
                }
                frame 3 {
                  w771 = TRUE
                  # "XYZ outside limit, move all"
                }
              }
              n436 = local write "XY Move"(w725) -> ()
              n437 = local write "Z Move"(w724) -> ()
            }
            frame "Move XYZ", "Move XY" {
              w805 = 2.0
              # "Initial XY stage positions"
              # "Check if move will go beyond ±2 µm of the original positions"
              n438 = case shown="True" TRUE {
                tunnel: w783 -> [_ w826]
                tunnel: [w824 w825] -> w778
                frame False {
                  n439 = local read "dxy (px)"() -> (w824:dbl[])
                }
                frame True {
                  # "Get XY Diff Values"
                  n440 = Array Subset(array=w826, index (row)=0 ("index"), length (row)=2 ("length"), index (col)=2 ("index")) -> (w827:dbl[][])  [unwired: 1 in]
                  n441 = Index Array(array=w827, index (col)=0 ("disabled index (col)")) -> (element=w825:dbl[])  [unwired: 1 in]
                }
              }
              n442 = Get Notifier Status(notifier=w822) -> (notifier out=w821:refnum<notifier>, current notification=w820:T8)  [unwired: 1 in, 3 out]
              n443 = Unbundle By Name(w820) -> ("Abort If Error"=w813:bool, "XY Stage Move Limit (µm)"=w816:dbl)
              n444 = Array Subset(array=w783, index (row)=0 ("index"), length (row)=2 ("length"), index (col)=3 ("index"), length (col)=1 ("length")) -> (w782:dbl[][])
              n445 = Index Array(array=w782, index (col)=0 ("disabled index (col)")) -> (element=w780:dbl[])  [unwired: 1 in]
              n446 = Equal?(x=4Pi_Obj_Lock_-_Actions."Move XYZ", y=w793) -> (x = y?=w791:bool)
              n447 = Build Array("X Update Scale Factor", "Y Update Scale Factor") -> (w774:dbl[])
              n448 = Select(t=4Pi_Obj_Lock_-_Actions."Move Z" ("x"), s=w791, f=4Pi_Obj_Lock_-_Actions."Update Plots") -> (s? t:f=w788:T6)
              n449 = Multiply(x=w778, y=w774) -> (x*y=w777:dbl[])
              n450 = call "Stages Messenger.vi"("Stage Notifier Name"=w797, "Actions"=Stage_Actions."Get Position") -> ("Stage Notifier Name (Dup)"=w796:string, "Positions"=w795:dbl[])  [unwired: 9 in, 3 out]
              n451 = call "4Pi Obj Lock - Rotate Flip XY.vi"("XY Amounts"=w777, "Flip XY"="Flip XY Axis", "Invert X"="Invert X Axis", "Invert Y"="Invert Y Axis") -> ("45° Rotated XY"=w779:dbl[])  [unwired: 11 in]
              n452 = Add(x=w795, y=w779) -> (x+y=w794:dbl[])
              n453 = Add(x=w780, y=w805) -> (x+y=w803:dbl[])
              n454 = Subtract(x=w780, y=w805) -> (x-y=w804:dbl[])
              n455 = Absolute Value(x=w779) -> (abs(x)=w815:dbl[])
              n456 = Greater?(x=w816, y=w815) -> (0:w814:bool[])
              n457 = In Range and Coerce(upper limit=w803, x=w794, lower limit=w804) -> (In Range?=w802:bool[])  [unwired: 1 out]
              n458 = And Array Elements(Boolean array=w814) -> (logical AND=w801:bool)
              n459 = And Array Elements(Boolean array=w802) -> (logical AND=w799:bool)
              n460 = And(x=w801, y=w799) -> (x .and. y?=w800:bool)
              n461 = Not(x=w800) -> (.not. x?=→"Move Limit Error":bool)
              n462 = case shown="True" w800 {
                tunnel: w779 -> [_ w842]
                tunnel: w813 -> [w836 _]
                tunnel: [w834 w839] -> w812
                tunnel: w796 -> [_ w841]
                tunnel: [dbl[] [-1.0, -1.0] ("Positions") w840] -> w810
                tunnel: w788 -> [w832 w839]
                frame False {
                  n463 = Select(t=4Pi_Obj_Lock_-_Actions."Abort" ("x"), s=w836, f=w832) -> (s? t:f=w834:T6)
                }
                frame True {
                  n464 = Wait (ms)(milliseconds to wait=u32 100) -> ()  [unwired: 1 out]
                  n465 = call "Stages Messenger.vi"("Stage Notifier Name"=w841, "Actions"=Stage_Actions."MVR", "Setpoint"=w842, "Axis"=bool[] [TRUE, TRUE], "Exit While Busy?"=FALSE) -> ("Positions"=w840:dbl[])  [unwired: 6 in, 4 out]
                }
              }
              n466 = Index Array(array=w810, index #1=0 ("index"), index #2=1 ("index")) -> (element #1=→"X Axis Position (µm)":dbl, element #2=→"Y Axis Position (µm)":dbl)
            }
            frame "Move Z" {
              w860 = 2.0 ("y")
              # "Initial Z stage position"
              n467 = Get Notifier Status(notifier=w878) -> (notifier out=w877:refnum<notifier>, current notification=w879:T8)  [unwired: 1 in, 3 out]
              n468 = case shown="True" TRUE {
                tunnel: [w881 w884] -> w872
                tunnel: w854 -> [_ w882]
                frame False {
                  n469 = local read "dz (µm)"() -> (w881:dbl)
                }
                frame True {
                  w883 = 0 ("disabled index (col)")
                  # "Get sx/sy Diff Value"
                  n470 = Array Subset(array=w882, index (row)=2 ("index"), length (row)=1 ("length"), index (col)=2 ("index"), length (col)=1 ("length")) -> (w886:dbl[][])
                  n471 = Index Array(array=w886, index (row)=w883, index (col)=w883) -> (element=w884:dbl)
                }
              }
              n472 = Index Array(array=w854, index (row)=2, index (col)=3 ("disabled index (col)")) -> (element=w851:dbl)
              n473 = Unbundle By Name(w879) -> ("Abort If Error"=w859:bool, "Z Stage Move Limit (µm)"=w864:dbl)
              n474 = Multiply(x=w872, y="Z Update Scale Factor") -> (x*y=w869:dbl)
              n475 = Add(x=w851, y=w860) -> (x+y=w866:dbl)
              n476 = Subtract(x=w851, y=w860) -> (x-y=w865:dbl)
              n477 = call "Stages Messenger.vi"("Stage Notifier Name"=w875, "Actions"=Stage_Actions."Get Position") -> ("Stage Notifier Name (Dup)"=w861:string, "Positions"=w873:dbl[])  [unwired: 9 in, 3 out]
              n478 = Negate(x=w869) -> (-x=w870:dbl)
              n479 = Select(t=w870, s="Invert Z Axis", f=w869) -> (s? t:f=w850:dbl)
              n480 = Index Array(array=w873, index=0) -> (element=w871:dbl)
              n481 = Absolute Value(x=w850) -> (abs(x)=w847:dbl)
              n482 = Add(x=w850, y=w871) -> (x+y=w867:dbl)
              n483 = Greater?(x=w864, y=w847) -> (0:w863:bool)
              n484 = Greater?(x=w847, y=0.002) -> (0:w845:bool)
              n485 = In Range and Coerce(upper limit=w866, x=w867, lower limit=w865) -> (In Range?=w862:bool)  [unwired: 1 out]
              n486 = And(x=w863, y=w862) -> (x .and. y?=w858:bool)
              n487 = Not(x=w858) -> (.not. x?=w857:bool)
              n488 = case shown="True" w858 {
                tunnel: w861 -> [_ w899]
                tunnel: w859 -> [w893 _]
                tunnel: w850 -> [_ w898]
                tunnel: [w892 4Pi_Obj_Lock_-_Actions."Update Plots" ("x")] -> w856
                tunnel: [-1.0 ("Position") w897] -> w855
                tunnel: w845 -> [_ w895]
                frame False {
                  n489 = Select(t=4Pi_Obj_Lock_-_Actions."Abort" ("x"), s=w893, f=4Pi_Obj_Lock_-_Actions."Update Plots") -> (s? t:f=w892:T6)
                }
                frame True {
                  n490 = case shown="True" w895 {
                    tunnel: w899 -> [w904 w909]
                    tunnel: w898 -> [_ w908]
                    tunnel: [w900 w906] -> w897
                    frame False {
                      n491 = call "Stages Messenger.vi"("Stage Notifier Name"=w904, "Actions"=Stage_Actions."Get Position") -> ("Positions"=w901:dbl[])  [unwired: 9 in, 4 out]
                      n492 = Index Array(array=w901, index=0) -> (element=w900:dbl)
                    }
                    frame True {
                      n493 = Build Array(w908) -> (w907:dbl[])
                      n494 = flat-sequence {
                        tunnel: w909 -> [w916]
                        tunnel: w907 -> [w915]
                        tunnel: [w911] -> w905
                        tunnel: [w919] -> w906
                        tunnel: w905 -> [w919]
                        frame #0 {
                          n495 = call "Stages Messenger.vi"("Stage Notifier Name"=w916, "Actions"=Stage_Actions."MVR", "Setpoint"=w915, "Axis"=bool[] [TRUE], "Exit While Busy?"=FALSE) -> ("Positions"=w913:dbl[])  [unwired: 6 in, 4 out]
                          n496 = Index Array(array=w913, index=0) -> (element=w911:dbl)
                        }
                        frame #1 {
                          n497 = Wait (ms)(milliseconds to wait=u32 150) -> ()  [unwired: 1 out]
                        }
                      }
                    }
                  }
                }
              }
              "Z Axis Position (µm)" <- w855
              n498 = local write "Move Limit Error"(w857) -> ()
            }
            frame "Update Plots" {
              (unwired) 0 ("index")
              # "Current Values"
              # "Target Values"
              n499 = Get Notifier Status(notifier=w1005) -> (notifier out=w1004:refnum<notifier>, current notification=w1006:T8)  [unwired: 1 in, 3 out]
              n500 = Unbundle By Name(w1006) -> ("Z Drift Threshold"=w997:dbl, "XY Drift Threshold"=w996:dbl)
              n501 = local read "X Axis Position (µm)"() -> (w991:dbl)
              n502 = local read "Y Axis Position (µm)"() -> (w990:dbl)
              n503 = local read "Z Axis Position (µm)"() -> (w989:dbl)
              n504 = Index Array(array=w986, index (col)=0 ("disabled index (col)")) -> (element=w983:dbl[])  [unwired: 1 in]
              n505 = Index Array(array=w986, index (col)=1 ("disabled index (col)")) -> (element=w984:dbl[])  [unwired: 1 in]
              n506 = Index Array(array=w986, index (col)=3 ("disabled index (col)")) -> (element=w987:dbl[])  [unwired: 1 in]
              n507 = Subtract(x=w984, y=w983) -> (x-y=w982:dbl[])
              n508 = local read "Measured Y Position cc (px)"() -> (w969:dbl)
              n509 = local read "Measured X Position cc (px)"() -> (w968:dbl)
              n510 = local read "Target X Position cc (px)"() -> (w970:dbl)
              n511 = local read "Target Y Position cc (px)"() -> (w971:dbl)
              n512 = Build Array(w991, w990, w989) -> (w988:dbl[])
              n513 = Index Array(array=w982, index #1=0 ("index"), index #2=1 ("index"), index #3=2 ("index")) -> (element #1=w967:dbl, element #2=w966:dbl, element #3=w924:dbl)
              n514 = Subtract(x=w988, y=w987) -> (x-y=w985:dbl[])
              n515 = Build Array(w967, w966) -> (w956:dbl[])
              n516 = Index Array(array=w985, index #1=0 ("index"), index #2=1 ("index"), index #3=2 ("index")) -> (element #1=w949:dbl, element #2=w948:dbl, element #3=w974:dbl)
              n517 = Build Array(w968, w969) -> (w972:dbl[])
              n518 = Build Array(w970, w971) -> (w973:dbl[])
              n519 = Build Array(w949, w948) -> (w942:dbl[])
              n520 = Subtract(x=w972, y=w973) -> (x-y=w965:dbl[])
              n521 = Square Root(x=2.0) -> (sqrt(x)=w944:dbl)
              n522 = Select(t=w956, s=FALSE, f=w965) -> (s? t:f=w963:dbl[])
              n523 = Divide(x=w942, y=w944) -> (x/y=w943:dbl[])
              n524 = Multiply(x="pixel size (µm)", y=w956) -> (x*y=w952:dbl[])
              n525 = Multiply(x="pixel size (µm)", y=w963) -> (x*y=w962:dbl[])
              n526 = Index Array(array=w943, index #1=0 ("index"), index #2=1 ("index")) -> (element #1=w941:dbl, element #2=w940:dbl)
              n527 = Index Array(array=w962, index #1=0 ("index"), index #2=1 ("index")) -> (element #1=w959:dbl, element #2=w958:dbl)
              n528 = Index Array(array=w952, index #1=0 ("index"), index #2=1 ("index")) -> (element #1=w951:dbl, element #2=w950:dbl)
              n529 = local read "Invert X Axis"() -> (w930:bool)
              n530 = Add(x=w941, y=w940) -> (x+y=w939:dbl)
              n531 = Subtract(x=w941, y=w940) -> (x-y=w933:dbl)
              n532 = Negate(x=w939) -> (-x=w934:dbl)
              n533 = local read "Invert Y Axis"() -> (w929:bool)
              n534 = Negate(x=w933) -> (-x=w937:dbl)
              n535 = Negate(x=w934) -> (-x=w938:dbl)
              n536 = local read "CC Max Value"() -> (w922:dbl)
              n537 = local read "Flip XY Axis"() -> (w931:bool)
              n538 = Select(t=w937, s=w929, f=w933) -> (s? t:f=w935:dbl)
              n539 = Select(t=w938, s=w930, f=w934) -> (s? t:f=w936:dbl)
              n540 = Bundle("CC Max Value"=w922) -> (→"CC Max":cluster{"CC Max Value":dbl})  [unwired: 1 in]
              n541 = Build Array(w936, w935) -> (w932:dbl[])
              n542 = case shown="True" w931 {
                tunnel: w932 -> [w1009 w1011]
                tunnel: [w1009 w1010] -> w927
                frame False {
                }
                frame True {
                  n543 = Reverse 1D Array(array=w1011) -> (reversed array=w1010:dbl[])
                }
              }
              n544 = Index Array(array=w927, index #2=1 ("index")) -> (element #1=w926:dbl, element #2=w925:dbl)  [unwired: 1 in]
              n545 = call "4Pi Obj Lock - 1 Values Organize Plot Data.vi"("Target 01"=0.0, "Value Limit"=w996, "Current 2"=w951, "Current 01"=w959, "Stage Pos"=w926) -> ("plot value"=→"X Target and Fit Position (µm)":T2)  [unwired: 10 in]
              n546 = Multiply(x=w924, y="Metric scale sx/sy") -> (x*y=w923:dbl)
              n547 = local read "Measured Z (µm)"() -> (w977:dbl)
              n548 = call "4Pi Obj Lock - 1 Values Organize Plot Data.vi"("Target 01"=0.0, "Value Limit"=w996, "Current 2"=w950, "Current 01"=w958, "Stage Pos"=w925) -> ("plot value"=→"Y Target and Fit Position (µm)":T2)  [unwired: 10 in]
              n549 = Select(t=w923, s=FALSE, f=w977) -> (s? t:f=w975:dbl)
              n550 = call "4Pi Obj Lock - 1 Values Organize Plot Data.vi"("Target 01"=0.0, "Value Limit"=w997, "Current 2"=w923, "Current 01"=w975, "Stage Pos"=w974) -> ("plot value"=→"Z Target and Fit Value (µm)":T2)  [unwired: 10 in]
            }
            frame "Delay" {
              n551 = Get Notifier Status(notifier=w1017) -> (notifier out=w1015:refnum<notifier>, current notification=w1018:T8)  [unwired: 1 in, 3 out]
              n552 = Unbundle By Name(w1018) -> ("Update Delay (ms)"=w1014:i32)
              n553 = while {
                tunnel: w1015 -> [w1030]
                tunnel: w1014 -> [w1027]
                tunnel: [w1023] -> w1013
                i -> [w1028]
                stop <- w1021 stop-if-true
                n554 = Get Notifier Status(notifier=w1030) -> (notifier out=w1023:refnum<notifier>, current notification=w1026:T8)  [unwired: 1 in, 3 out]
                n555 = Greater Or Equal?(x=w1028, y=w1027) -> (x >= y?=w1022:bool)
                n556 = Wait (ms)(milliseconds to wait=u32 1) -> ()  [unwired: 1 out]
                n557 = Unbundle By Name(w1026) -> ("Actions"=w1025:T6)
                n558 = Equal?(x=w1025, y=4Pi_Obj_Lock_-_Actions."Abort") -> (x = y?=w1020:bool)
                n559 = Or(x=w1020, y=w1022) -> (x .or. y?=w1021:bool)
              }
            }
            frame "Abort" {
              w1034 = 0.0 ("Target X Position (px)")
              n560 = Get Notifier Status(notifier=w1040) -> (notifier out=w1044:refnum<notifier>, current notification=w1043:T8)  [unwired: 1 in, 3 out]
              n561 = call "Camera Messenger.vi"("Notifier Name"=w1032, "General Camera Actions"=Generic_Camera_Actions."Abort") -> ()  [unwired: 8 in, 6 out]
              n562 = Bundle By Name(cluster=w1043, "Running?"=FALSE, "Actions"=4Pi_Obj_Lock_-_Actions."Exit Loop") -> (w1041:T8)
              n563 = Send Notification(notification=w1041, notifier=w1044) -> (notifier out=w1039:refnum<notifier>)  [unwired: 1 in, 1 out]
              n564 = local write "Start Lock"(FALSE ("Start Lock")) -> ()
              n565 = local write "Measured X Position (px)"(w1034) -> ()
              n566 = local write "Measured Y Position (px)"(w1034) -> ()
              n567 = local write "Target X Position (px)"(w1034) -> ()
              n568 = local write "Target Y Position (px)"(w1034) -> ()
              n569 = local write "Measured sx/sy"(w1034) -> ()
              n570 = local write "Target sx/sy"(w1034) -> ()
            }
            frame "Exit Loop" {
            }
            frame "Quit" {
              n571 = Get Notifier Status(notifier=w1050) -> (notifier out=w1049:refnum<notifier>, current notification=w1057:T8)  [unwired: 1 in, 3 out]
              n572 = Unbundle By Name(w1057) -> ("Ref Stack (SGL)"=w1056:T9[], "Cur Image (SGL)"=w1055:T9, "Tmp Image FFT (CSG)"=w1054:T9[], "CC Image (SGL)"=w1053:T9, "Ref FFT Stack (CSG)"=w1051:T9[])
              n573 = Release Notifier(notifier=w1049, force destroy? (F)=TRUE) -> ()  [unwired: 1 in, 3 out]
              n574 = Build Array (concatenate)(w1056, w1055, w1054, w1053, w1051) -> (w1052:T9[])
              n575 = for {
                tunnel: w1052 -> [w1062] mode=indexing
                n576 = call "IMAQ Dispose"("Image"=w1062) -> ()  [unwired: 5 in, 1 out]
              }
            }
          }
          n577 = Get Notifier Status(notifier=w234) -> (current notification=w233:T8, error out=w228:errorcluster)  [unwired: 1 in, 3 out]
          n578 = Unbundle By Name(w233) -> ("Actions"=w232:T6)
          n579 = Unbundle By Name(w228) -> ("status"=w226:bool)
          n580 = Equal?(x=w231, y=w232) -> (x = y?=w227:bool)
          n581 = Or(x=w227, y=w226) -> (x .or. y?=w225:bool)
          n582 = Select(t=w231, s=w225, f=w230) -> (s? t:f=w229:T6)
        }
      }
      n583 = local write "Quit"(w208) -> ()
    }
    frame Error {
    }
  }
  n584 = control-ref of="This VI"() -> (w87:refnum<vi>)
  n585 = property class="VI"(reference=w87) -> (reference out=w96:refnum<vi>, "Panel"=w88:refnum<vi>)  [unwired: 1 in, 1 out]
  n586 = property class="Pnl"(reference=w88) -> ("Decos[]"=w86:refnum<vi>[], "Panes[]"=w92:refnum<vi>[])  [unwired: 1 in, 2 out]
  n587 = Array Size(array=w86) -> (size(s)=w84:i32)
  n588 = Decrement(x=w84) -> (x-1=w85:i32)
  n589 = Index Array(array=w92, index=0) -> (element=w91:refnum<vi>)
  n590 = Index Array(array=w86, index=w85) -> (element=w94:refnum<vi>)
  n591 = property class="VI"(reference=w96) -> (reference out=w98:refnum<vi>, "Front Panel.PanelBounds"=w99:T22)  [unwired: 1 in, 1 out]
  n592 = property class="Decor"(reference=w94) -> ("Bounds"=w97:T23)  [unwired: 1 in, 2 out]
  n593 = property class="Pane"(reference=w91, "Origin"=T11 {"Horizontal"=0, "Vertical"=0}, "HorizScrollbarVisibility"=w95, "VertScrollbarVisibility"=w95) -> ()  [unwired: 1 in, 2 out]
  n594 = Unbundle By Name(w97) -> ("Width"=w102:u32, "Height"=w105:u32)
  n595 = control-ref of="Quit"() -> (w89:refnum<vi>)
  n596 = To Word Integer(number=w102) -> (16bit integer=w104:i16)
  n597 = To Word Integer(number=w105) -> ()  [unwired: 1 out]
  n598 = property class="Bool (strict)"(reference=w89) -> ("Height"=w107:u32, "Top"=w108:i32)  [unwired: 1 in, 2 out]
  n599 = Unbundle By Name(w99) -> ("Left"=w101:i16, "Top"=w112:i16)
  n600 = To Word Integer(number=w107) -> (16bit integer=w110:i16)
  n601 = To Word Integer(number=w108) -> (16bit integer=w111:i16)
  n602 = Add(x=w101, y=w104) -> (x+y=w103:i16)
  n603 = Compound Arithmetic op=ADD(w112, w110, w111, i16 12 ("y")) -> (w106:i16)
  n604 = Bundle By Name(cluster=w99, "Right"=w103, "Bottom"=w106) -> (w100:T22)
  n605 = property class="VI"(reference=w98, "Front Panel.PanelBounds"=w100) -> ()  [unwired: 1 in, 2 out]
